vi "Doktorarbeit_Cornelius_1.8.vi"(0 "Heizer":refnum<visa-resource-name>="COM1", 1 "Setpoint\n START":bool, 2 "Write to File":bool, 3 "SP 1 shall be (°C)":dbl=20.0 min=0.0 max=999.0, 4 "Intervall (s)":u32=1 max=600, 5 "Write/\nRead":bool=TRUE, 6 "Delay (ms)":u32=500 min=100 max=600000, 7 "Auto Tune":bool, 9 "Standby":bool, 11 "Reset\nSTOPP":bool, 12 "ON":bool=TRUE caption="OFF", 13 "Get Values":bool, 15 "File Path":path) -> (8 "(°C)":dbl format="%#.3f", 14 "SP 1 is (°C)":dbl)   [LabVIEW 2010]
doc: "1. Verwendung\n\nDas Programm dient der Steuerung und Abfrage des Thermocontrollers I3252 und dem Auslesen von zwei VC 840 Messgeräten und einem Druckmessgerät Pfeiffer Single Gauge. \nDie Messgeräte werden Standardmäßig ausgelesen und erst nach Betätigung des Schalters \"Write to File\" in einer Textdatei abgespeichert. Das Eingabefeld \"Intervall\" legt den Abstand der Messpunkte fest.\nDer Setpoint für den Thermocontroller wird erst nach Betätigung des Tasters \"Setpoint START\" übernommen und angesteuert. Er wird ind den EEPROM des Gerätes geschrieben. Die Regelung kann mit Hilfe des Schalters \"Standby\" unterbrochen werden. Durch den Taster \"Reset STOPP\" kann der Setpoint aus dem EEPROM gelöscht werden.\nDie Eingabeflächen \"Constant\" und \"Thickness\" dienen der Berechnung des spezifischen Widerstands.\nDie Eingabeflächen \"User\" und \"Sample\" werden in den Header der Textdatei übernommen.\nDer Indikator \"File Path\" zeigt den aktuellen Speicherort der Textdatei an. Dieser wird nach ausschalten des Schalters \"Write to File\" gelöscht. Bei erneuten Schreiben muss ein neuer Speicherort gewählt werden. Bei Wahl desselben Speicherorts werden sämtliche bereits gespeicherte Daten gelöscht.\n\n\n2. Erläuterungen zum Blockdiagramm\n2.1 äußere Sequenz\nDie äußerte Sequenz besteht aus fünf Frames. Der erste dient der Initialisierung der Ports. Der zweite dient als Verzögerung um dem Programm genug Zeit zu geben die Ports zu öffnen. Jedoch senden die beiden VC 840 bereits Informationen an den Computer die in einem Puffer zwischengespeichert werden. Im dritten Frame wird dieser Puffer geleert. Somit kommt es zu keinem Framing Error. Desweiteren wird in diesem Frame die Startzeit der Messungen genommen. Im vierten Frame wird die eigentliche Messung und Verarbeitung der Daten durchgeführt. Die while-Schleife wird nur durch Auftreten eines Fehlers oder durch Betätigung des Stopbuttons auf dem Front Panel in der oberen linken Ecke unterbrochen. Im fünften und letzten Frame werden die Ports wieder geschlossen und beim Auftreten eines Fehlers wird das Programm automatisch gestoppt. Falls kein Fehler auftritt wird die Sequenz von vorne abgearbeitet.\n\n2.2 while-Schleife und innere Sequenz\n2.2.1 \"Event Structure\"\n2.2.1.1 Allgemein\nDer erste Frame beinhaltet ein \"Event Structure\". Dieser reagiert auf insgesamt elf verschiedene Ereignisse. Falls keines dieser Ereignisse auftreten sollte, warte die Struktur eine Millisekunde bevor die \"Event Structure\" verlassen wird. Die übrigen Ereignisse treten ein, wenn der entsprechende Kontroller eine Werteänderung erfährt.\n\n2.2.1.2 Event: Setpoint\nDieser Case besteht von außen nach innen aus einer Stacked Sequence, einer for-Loop und einer Flat Sequence die wiederum zwei \"Case Structures\" enthält. Als erstes wird bei dem Schalter \"Setpoint START\" der Blinkmodus aktiviert und bei dem Schalter \"Read Temperature\" deaktiviert. Danach folgt das eigentliche setzen des Temperatursollwerts. In der ersten Iteration wird dem Controller I3252 ein Schreibbefehl gesendet. Theoretisch kann der Setpoint in den RAM oder in den EEPROM geschrieben werden. Diese Auswahl erfolgt mit Hilfe des Schalters \"RAM\". Da das Schreiben in den RAM -Speicher aber aus diversen Gründen nicht erwünscht ist, wurde es nicht implementiert. Eine nachträgliche Implementierung ist aber leicht möglich, in dem die untere String-Konstante \"*P012\" durch \"*W012\" ersetzt wird. An diesem Befehl wird eine fünfstellige Hexadezimalzahl angehängt, die den Sollwert wiedergibt. Der Sollwert wird vorher mit zehn multipliziert, da das Komma standardmäßig nach der ersten Ziffer festgesetzt wurde (Bsp.: 800 wird gesendet um 80 einzustellen). Dieser Befehlsstrang wird an das Gerät mittels des SubVIs \"Comm_Interface\", auf welches später noch näher eingegangen wird, weitergegeben. Der durch das Gerät zurückgegebene String wird nicht verarbeitet.\nDie zweite Iteration dient dem Auslesen des eingestellten Sollwertes. Wahlweise kann der RAM- oder der EEPROM-Speicher ausgelesen werden. Die eigentliche Verarbeitung des Ausgabestrings erfolgt durch das SubVI \"Edit Setpoint\".\nDie Implementierung zur Einstellung des zweiten Setpoints erfolgt durch kopieren der ersten beiden Fälle und ersetzen der \"1\" im Befehf durch eine \"2\" (Bsp.: \"*P012\" zu \"*P022\"). Es darf aber nicht vergessen werden, dass dann ebenfalls die Anzahl der Iterationen angepasst werden muss.\nAls letztes wird der Blinkmodus des Schalters \"Setpoint START\" wieder deaktiviert.\n\n2.2.1.3 Event: Standby\nDieses Ereignis aktiviert bzw. deaktiviert als erstes den Blinckmodus des entsprechenden Schalters und sendet danach den Befehl zum aktivieren (\"*D03\") oder zum deaktivieren (\"*E03\") des Standbymodus an den Thermocontroller.\n\n2.2.1.4 Event: Set Command \nDer in das Feld \"Command shall be\" eingegebene Befehl wird an den Thermocontroller übermittlet. Die korrekte Form des Befehls ist im \"Communication Manuel\" nachzuschlagen. Das \"*\"-Zeichen wurde allerdings schon implementiert und muss somit nicht mit eingegeben werden.\n\n2.2.1.5 Event: Reset\nIn der ersten Iteration wird der Reset-Befehl an den Thermocontroller gesendet. In Folge wird der gesamte EEPROM-Speicher gelöscht. Deshalb wird in der zweiten Iteration der Setpoint aktualisiert. Dieser Befehl hat keinen Einfluss auf den RAM-Speicher. Die anschließende Wartezeit ist auf vier Sekunden festgesetzt und wurde empirisch ermittelt. Diese Zeit benötigt das Gerät um den Reset durchzuführen und für die Kommunikation wieder zur Verfügung zu stehen.\n\n2.2.1.6 Event: Auto Tune\nEs ist festgeschrieben, dass der Setpoint für die \"Auto Tune\"-Funktion wenigstens 20°C über der aktuellen Temperatur liegt. Deshalb wird zunächst der aktuelle Temperaturwert ausgelesen. Im zweiten Schritt werden zu diesem Wert zwanzig addiert und der Setpoint wird in den RAM-Speicher geschrieben. Das Schreiben in diesen Speicher ist nötig, da die \"Auto Tune\"-Funktion\" erst nach einem Reset startet. Im dritten Schritt wird der eigentliche Befehl für den \"Auto Tune\" gesendet (siehe dazu \"Communication Manuel\" S.27). Als vierte und letzte Iteration der for-Schleife folgt der bereits erwähnte Reset-Befehl. Der Temperatursollwert, der im RAM-Speicher eingetragen ist, muss zum Schluss wieder auf 0°C gesetzt werden. Die Zeit für die Ausführung des \"Auto Tune\"-Befehls wurde empirisch ermittelt und 45 s festgesetzt.\n\n2.2.1.7 Event: Write LOW/HI\nDieses Ereignis setzt die am Analogausgang anliegende Spannung fest. Normalerweise beträgt dieser Spannungswert 0-10 V. Das angeschlossene Netzteil verträgt aber maximal nur 2,3 V. Aus diesem Grund wird der \"%HIGH\" auf 23 gesetzt. Somit beträgt die maximal anliegende Spannung nur noch 23% von der maximal möglichen, d.h 2,3V. Ein niedrigerer Wert ist jederzeit möglich, genauso wie ein höherer für den Parameter \"%LOW\". Diese werden zunächst nacheinander in den RAM-Speicher geschrieben und anschließend wieder ausgelesen.\n\n2.2.1.8 Event: Set PID\nDie Werte für den PID-Regler können sowohl mit Hilfe der \"Auto Tune\"-Funktion, als auch manuell eingestellt werden. Es wird wiederum zwischen dem Schreiben in den RAM- und dem EEPROM-Speicher unterschieden. Zunächst werden die Werte für \"P\", \"I\" und \"D\", in dieser Reihenfolge, gesetzt und danach die aktuellen Werte ausgelesen.\n\n2.2.1.9 Event: Get Values\nDieses Ereignis hat zur Folge, dass die Werte für \"P\", \"I\", \"D\", \"%LOW\", \"%HIGH\" und des Setpoints wahlweise aus dem RAM- oder EEPROM-Speicher gelesen werden. Die aktuellen Werte werden nicht nur in die entsprechenden Anzeigefelder übernommen, sondern auch in die entsprechenden Eingabefelder, mit Ausnahme des Temperatursollwerts. \n\n2.2.1.10 Event: RAM\nPrinzipiell kann zwischen dem Schreiben in den RAM- oder EEPROM-Speicher des Thermocontrollers gewählt werden. Die entsprechende Schalterposition auf dem Frontpanel zeigt den aktuell verwendeten Speicher an. Die Anzeigewerte werden bei jedem Umschalten aktualisiert und sind im entsprechenden Speicher eingetragen. Die Implementierung ist identisch mit der des Ereignisses \"Get Values\". Es gilt zu beachten, dass die Werte für \"%LOW\" und \"%HIGH\" nur in den RAM-Speicher geschrieben werden können und somit auch nur aus diesem ausgelesen werden können.\n\n2.2.1.11 Event: Set Gauge to Zero\nMit Hilfe der SubVIs \"Get Pressure\" und \"Offset Display\" werden die Werte für den alten und den neuen Offset und der durch den zweiten Drucksensor ermittelt Druck ermittelt. \n\n2.2.1.12 Event: Write to File\nSollte der Schalter \"Write to File\" aktiviert werden, d.h. Schalterposition oben, so wird zunächst durch das SubVI \"Header\" ein Header für die unter \"File Path\" definierte Datei angelegt. Alle Werte, die bereits in der entsprechenden Datei stehen, werden dabei gelöscht.\n\n2.2.2 \"Timed Structures\"\nIm dritten Frame der inneren Sequenz werden die Werte für Zeitpunkt, Temperatur, Spannung, Strom und Druck ermittelt. Damit die Werte zum gleichen Zeitpunkt aufgenommen werden, werden \"Timed Sequences\" eingesetzt. Mit dem entsprechenden Schalter auf dem Front Panel unter dem Tab \"Settings\" kann gewählt werden, ob das entsprechende Gerät ausgelesen werden soll oder nicht. Die einzelnen Sequenzen werden parallel abgearbeitet, womit die Prozesszeit von diesem Frame durch der zeitintensivsten Sequenz abhängt. Dies ist in aller Regel das Auslesen der Temperatur, da ein \"Delay\" von 500 ms oder größer benötigt wird, um den Controller ordentlich ansprechen zu können.\nDie Systemzeit wird durch das SubVI \"System Time in Seconds\" in Sekunden umgerechnet und der in dem Parameter \"Starttime\" gespeicherte Wert wird abgezogen. Somit werden die Sekunden seit dem Start des Programms gezählt.\n\n2.2.3 restlichen Frames\nIm zweiten Frame wird das Intervall zwischen den einzelnen Messwerten festgelegt. Dabei wird der Wert des Parameters \"Delay\" abgezogen. Dieser Wert beträgt im Normalfall 500 ms und ist somit nicht vernachlääsigbar.\nDer Vierte Frame beinhaltet die Umrechnung des Temperatur-Strings in einen Temperaturwert durch das SubVI \"Edit Tmperature\", die Berechnung des spezifischen Widerstands durch das SubVI \"Resistivity Calculation\" und die Überprüfung des Druckwerts. Auch werden die neu gewonnen Werte in das entsprechende Shift-Register übernommen. Falls der Druckwert einen in dem Parameter \"Pressure Limit (mbar)\" festgelegten Grenzwert überschreiten sollte, wird der Thermocontroller automatisch in den Standby-Modus versetzt. Des Weiteren wird der Schalter \"Standby\" solange gesperrt, wie der Druck oberhalb des Grenzwertes liegt. Wenn der Druck wieder unter den Grenzwert gesunken ist, wird der Standby-Befehl nicht automatisch aufgehoben, sondern muss vom Benutzer durch Betätigung des entsprechenden Schalters gegeben werden.\nIm fünften Frame werden die Diagramme erstellt. Dabei wird jedes Mal von neuem das gesamte Shift-Register als Graph dargestellt. Weiterhin werden die Messwerte in ein 1D-Array geschrieben.\nDer sechste und letzte Frame beinhaltet den eigentlich Schreibvorgang der Messwerte in eine Textdatei und die Überprüfung ob ein Fehler vorliegt.\n\n2.3 SubVIs\n2.3.1 Allgemein\nDie SubVIs für die Messgeräte VC840 und das Druckmessgerät wurden aus anderen Quellen übernommen. \n\n2.3.2 \"Header\"\nIn den Header wird zunächst das aktuelle Datum und die aktuelle Zeit übernommen. Die ausgewählte Datei wird dabei überschrieben. Danach wird der Name des Benutzers und der Probe übernommen. Zum Schluss werden die Einheiten in einer Reihe, durch einen Tabulator getrennt, in den Header geschrieben.\n\n2.3.3 \"I3252 Comm Interface\"\nDieses VI stellt die Kommunikation mit dem Thermocontroller her und gibt den Ausgabe-String zurück.\n\n2.3.4 \"I3252 Edit Setpoint\"\nIm Ausgabe-String vom Thermocontroller ist an der vierten Stelle die Stelle des Dezimalpunktes verschlüsselt. Dieses Hexadezimalzahl wird herausgefiltert und an ein \"ENUM Controller\" übergeben. Dieser weist der Hexadezimalzahl eine Nummer zu, mit welcher ein Wert aus einem Array entnommen wird. Dieser Wert dient als Quotient. Der tatsächliche Wert kann somit errechnet werden.\n\n2.3.5 \"I3252 Edit Temperature\"\nDer Temperatur-String, der vom Thermocontroller zurückgegeben wird, wird in eine Dezimalzahl umgewandelt. Manchmal kommt es aus zu Dropouts, die durch dieses Programm herausgefiltert werden. Der letzte Wert wird dabei in einer \"Feedback Node\" gehalten unter der Annahme, dass sich der Temperaturwert nicht sprunghaft ändert.\n\n2.3.6 \"Resistivity Calculation\"\nDer spezifische Widerstand wird nach folgender Formel ausgerechnet. Dabei entspricht t der Dicke der Probe und C ist eine Konstante.\nrho=C*pi*t*U/(ln( 2)*I)\n\n2.3.7 \"System Time in Seconds\"\nZunächst wird die aktuelle Systemzeit ausgelesen. Danach wird diese in Stunden, Minuten und Sekunden aufgeteilt, alles in Sekunden umgerechnet und letztendlich addiert."
uses:
  <vilib>/Platform/TimedLoop/XDataNode/XDataNode.xnode
  <vilib>/Platform/TimedLoop/XDataNode/timing_clust.ctl
  <vilib>/Platform/TimedLoop/XDataNode/nitl_modes.ctl
  <vilib>/Platform/TimedLoop/XDataNode/wakeup.ctl
  <vilib>/Instr/_visa.llb/VISA Configure Serial Port (Instr).vi
  <vilib>/Platform/TimedLoop/scheduler/LVUserAPI/_suppVIs/Create_1kHz_TSource.vi
  <vilib>/Utility/file.llb/Write To Spreadsheet File (DBL).vi
  <vilib>/Platform/TimedLoop/XDataNode/XDNodeRunTimeDep.lvlib
  Labview 8 Tutorial/Dual Gauge/Dual Gauge.lvlib
panel:
  in  "Delay (ms) 2":u32=500 min=100 max=600000
  in  "Write/\nRead 2":bool=TRUE
  in  "Flow Control 2":u16(ring) items=["None"=0, "XON/XOFF"=1, "RTS/CTS"=2, "DTR/DSR"=4]
  in  "Stop Bits 2":u16(ring)=10 items=["1.0"=10, "1.5"=15, "2.0"=20]
  in  "Parity 2":u16(ring)=1 items=["None", "Odd", "Even", "Mark", "Space"]
  in  "Data Bits 2":u16=7 min=5 max=8 step=1
  in  "Baud Rate 2":u32=9600
  in  "Heizer 2":refnum<visa-resource-name>="COM1"
  out "appended array":dbl[](array[numeric])
  in  "Tab Control":T1(tab)
  out "Pirani (VVP1 Scroll)":cluster{dbl[], dbl[]}(graph)
  in  "Thickness (nm)":dbl min=0.0
  in  "Constant":dbl=4.532 min=0.0 max=5.0
  in  "Sample":string
  in  "User":string
  out "Thermocouple (Sample holder 1)":cluster{dbl[], dbl[]}(graph)
  out "current time (s)":dbl
  out "data logger intervall (s)":dbl
  out "loop time (s)":dbl
  in  "stop":bool
  out "CMR275 Baratron":cluster{dbl[], dbl[]}(graph)
  out "Pressure Baratron 2":dbl format="%#_4e"
  out "PKR251 FullRange":cluster{dbl[], dbl[]}(graph)
  out "Pressure FullRange 2":dbl format="%#_3e"
  out "Pressure Pirani 2":dbl format="%#_3e"
  out "Pressure OpenPort":cluster{dbl[], dbl[]}(graph)
  out "Pressure OpenPort2":dbl caption="current"
  out "status 2":bool caption="Status"
  out "code 2":i32 caption="Code"
  out "code":i32 caption="Code"
  out "status":bool caption="Status"
  in  "Set Gauge to Zero":bool
  out "Status Gauge 1#2":i32(ring) items=["data OK", "underrange", "overrange", "sensor error", "sensor off", "no sensor", "ID error"]
  out "Pressure Gauge 1#2":dbl format="%.3e"
  out "Pressure Gauge 1#1":dbl format="%.3e"
  out "Status Gauge 1#1":i32(ring) items=["data OK", "underrange", "overrange", "sensor error", "sensor off", "no sensor", "ID error"]
  in  "TPG 1 COM":refnum<visa-resource-name>="COM5"
  in  "Pressure Limit (mbar)":dbl=1.0 min=0.0 max=1100.0
  out "Current Offset (mbar)":dbl
  in  "ON (TPG 2)":bool=TRUE caption="OFF"
  in  "ON (TPG 1)":bool=TRUE caption="OFF"
  in  "ON":bool caption="OFF"
  in  "VC 840 2":refnum<visa-resource-name>="COM7"
  out "Reading 2":dbl format="%_4f"
  out "Mode 2":enum16{"?", "Diode", "Beep", "DC", "AC"}(ring)
  out "Unit 2":string
  in  "VC 840 1":refnum<visa-resource-name>="COM7"
  out "Reading 1":dbl format="%_4f"
  out "Mode 1":enum16{"?", "Diode", "Beep", "DC", "AC"}(ring)
  out "Unit 1":string
  out "Status 1":T2
  out "Status 2":T2
  in  "ON":bool caption="OFF"
  out "% HIGH Istwert":u32
  out "% LOW Istwert":u32
  in  "% High Sollwert":u32=23 max=24
  in  "% LOW Sollwert":u32 max=25
  in  "RAM":bool=TRUE caption="EEPROM"
  out "D (Rate) IstWert":u32
  out "I ( Reset1) Istwert":u32
  out "P (PB1) Istwert":u32 caption="actual value"
  in  "D (Rate) Sollwert":u32 max=3999
  in  "I ( Reset1) Sollwert":u32 max=3999
  in  "P (PB1) Sollwert":u32 caption="set value" max=9999
  in  "Set Command":bool
  in  "Set PID":bool
  in  "Write LOW/HI":bool
  in  "Flow Control":u16(ring) items=["None"=0, "XON/XOFF"=1, "RTS/CTS"=2, "DTR/DSR"=4]
  in  "Stop Bits":u16(ring)=10 items=["1.0"=10, "1.5"=15, "2.0"=20]
  in  "Parity":u16(ring)=1 items=["None", "Odd", "Even", "Mark", "Space"]
  in  "Data Bits":u16=7 min=5 max=8 step=1
  in  "Baud Rate":u32=9600
  out "Command output":string
  in  "Command input":string
  in  "TPG 2 COM":refnum<visa-resource-name>="COM6"
  out "Pressure Gauge 2#2":dbl format="%.3e"
  out "Pressure Gauge 2#1":dbl format="%.3e"
  out "Status Gauge 2#2":i32(ring) items=["data OK", "underrange", "overrange", "sensor error", "sensor off", "no sensor", "ID error"]
  out "Status Gauge 2#1":i32(ring) items=["data OK", "underrange", "overrange", "sensor error", "sensor off", "no sensor", "ID error"]
  out "Current":cluster{dbl[], dbl[]}(graph)
  out "Voltage":cluster{dbl[], dbl[]}(graph)
  out "Voltage (V)":dbl format="%.4e"
  out "Current (A)":dbl format="%.4e"
  out "Resistivity":cluster{dbl[], dbl[]}(graph)
  out "Resistivity (Ohm*cm)":dbl format="%.3e"
  # "mbar"
  # "mbar"
  # "mbar"
  # "mbar"
  # "Pressure Measurement \n(Pfeiffer TPG261)"
  # "PID Controller (Omega Newport i3252)"
  # "PID Controller (Omega Newport i3252)"
  # "limit (mbar)"
  # "Multimeter\n#1 (VC 840)"
  # "Multimeter\n#2 (VC 840)"
  # "P"
  # "I"
  # "D"
  # "% Low"
  # "% High"
  # "Authors:  Daniel Schuster (sir-dan@web.de)\n                 Steffen Cornelius (s.cornelius@hzdr.de)\n                 Nico Spahn (x)\n\n                 premade SubVIs for readout of Pfeiffer gauge and VC840 Multimeters were used\n                 SubVI \"I3252_Comm_Interface\" is based on a modified Labview example\n\nRelease:  v1.0    \n\nVersion History:\n\nv1.1  -    28.06.2011\n             - Format des Files geändert von %.3f auf %g\n             - maximale Eingabewerte für PID begrenzt\nv1.2  -    12.07.2011\n             - Anzeige p,rho, U, V auf Scientific geändert\n             - y-Achse p,rho auf Log geändert\n             - numerische Zeitanzeige hinzugefügt\n             - 4PP Constant: pi/ln(2)=4,532 set as the default value\nv1.3  -    25.07.2011\n             - Zeitvariable auf EXT geändert, um Sprünge in Diagrammen loszuwerden\nv1.4  -   27.07.2011\n             - ALLE Variablen auf DBL zurückgesetzt wegen Formatierungsproblem im File\n             - Zeitberechnung neu gemacht (Tick count differenzen) -> Zeitsprünge korrigiert ?\n             - Delay/Intervall überarbeitet\nv1.5  -   05.12.2012\n                - Austausch der alten Pfeifer SubvIs durch neue -> nun alle 4 Kanäle des DualGauge\n                                                                                                         Controllers gleichzeitig auslesbar\n                - neue Pfeiffer SubVIs verwendet in Druckwertauslesung und Offset Berechnung des Baratron\n                  Druckes (COM5 Sensor1)\n                - Neuarragement des GUI -> FullRange und Baratron neben Temperatur auf Haupseite zu sehen\n                                                                   Pirani und OpenPort auf Meas.2 zu sehen\n                                                                   Diagnose Seite umfasst nun auch Widerstandsdiagramm\n                - Änderungen der Settingseite -> nun alle 4 Drucksensoren mit aktuellem Messwert und Gerätestatus\n                                                                           zu sehen\n                - The readout of the PID-Temperature Controller and the VC840 Multimeters was not modified\nv1.73  -  18.10.2013\n                - Layout Änderungen\nv.1.8   -  19.01.2014\n                - Änderung Layout Settings Tab\n                - Trennung der beiden TPG Dual Gauge Controls\n                -"
  # "Version 1.73    - last change 18.10.2013"
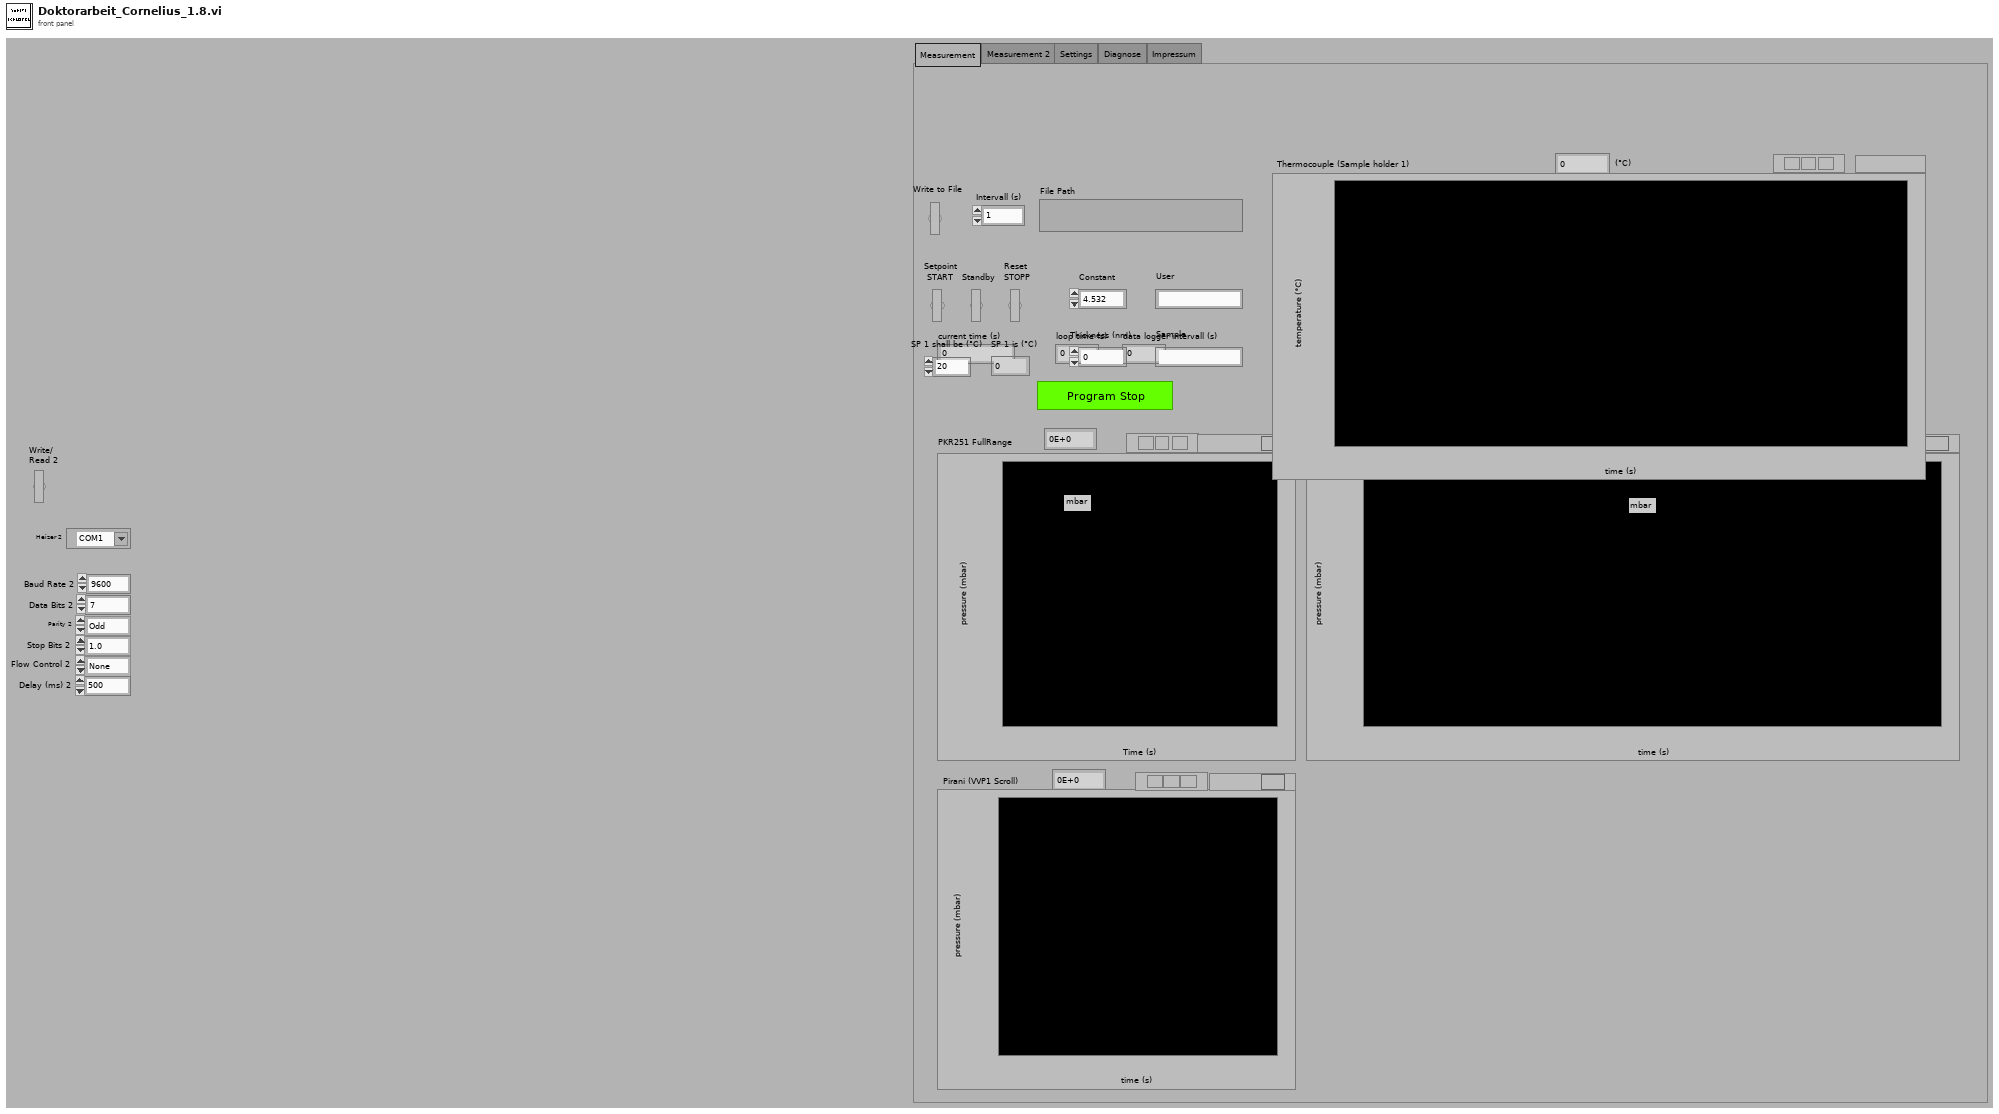
[diagram p1: front panel]
types:
  T1 = enum32{"Measurement", "Measurement 2", "Settings", "Diagnose", "Impressum"}
  T2 = cluster{"Low Bat":bool, "Auto":bool, "Delta":bool, "Hold":bool, "RS232":bool}
  T3 = typedef "XDNodeRunTimeDep.lvlib/timing_clust.ctl" = cluster{"Expected End [f-1]":u64, "Actual End [f-1]":u64, "Finished Late? [f-1]":bool, "Expected End [i-1]":u64, "Actual End [i-1]":u64, "Finished Late? [i-1]":bool, "Expected Start [i]":u64, "Actual Start [i]":u64, "Expected Start [f]":u64, "Actual Start [f]":u64, "Source Name":string, "Structure Name":string, "Period":i64, "Deadline":i64, "Offset":i64, "Start":i64, "Priority":i32, "Timeout":i32, "Mode":T4, "Wakeup Reason":T5, "Error":errorcluster, "Source Type":string, "Secondary Source Type":string, "Global End Time":u64, "Global Start Time":u64, "Frame Duration":u64, "Iteration Duration":u64, "Assigned CPU":i32, "I/O Scan Engine Mode":u32}
  T4 = typedef "XDNodeRunTimeDep.lvlib/nitl_modes.ctl" = enum32{"No Change", "Process missed periods, maintain original phase", "Discard missed periods, maintain original phase", "Process missed periods, ignore original phase", "Discard missed periods, ignore original phase"}
  T5 = typedef "XDNodeRunTimeDep.lvlib/wakeup.ctl" = enum32{"Normal", "Aborted", "Asynchronous wakeup", "Timing source error", "Timed loop error", "Timeout"}
  T6 = enum8{"Enabled", "Disabled", "Disabled and Grayed Out"}
  T7 = cluster{"VISA resource name out":refnum<visa-resource-name>, "error out":errorcluster, "Delay (ms)":u32, "Write/\nRead":bool}
  T8 = cluster{"TPG 2 COM":refnum<visa-resource-name>, "error out":errorcluster}
  T9 = cluster{"COM out":refnum<visa-resource-name>, "Cluster (Ausgang)":errorcluster}
  T10 = cluster{"Pressure Gauge#1":dbl, "Pressure Gauge#2":dbl}
  T11 = cluster{"TPG 1 COM":refnum<visa-resource-name>, "error out":errorcluster}
  T12 = cluster{"COM out":refnum<visa-resource-name>, "error out":errorcluster, "COM out":refnum<visa-resource-name>, "error out":errorcluster}
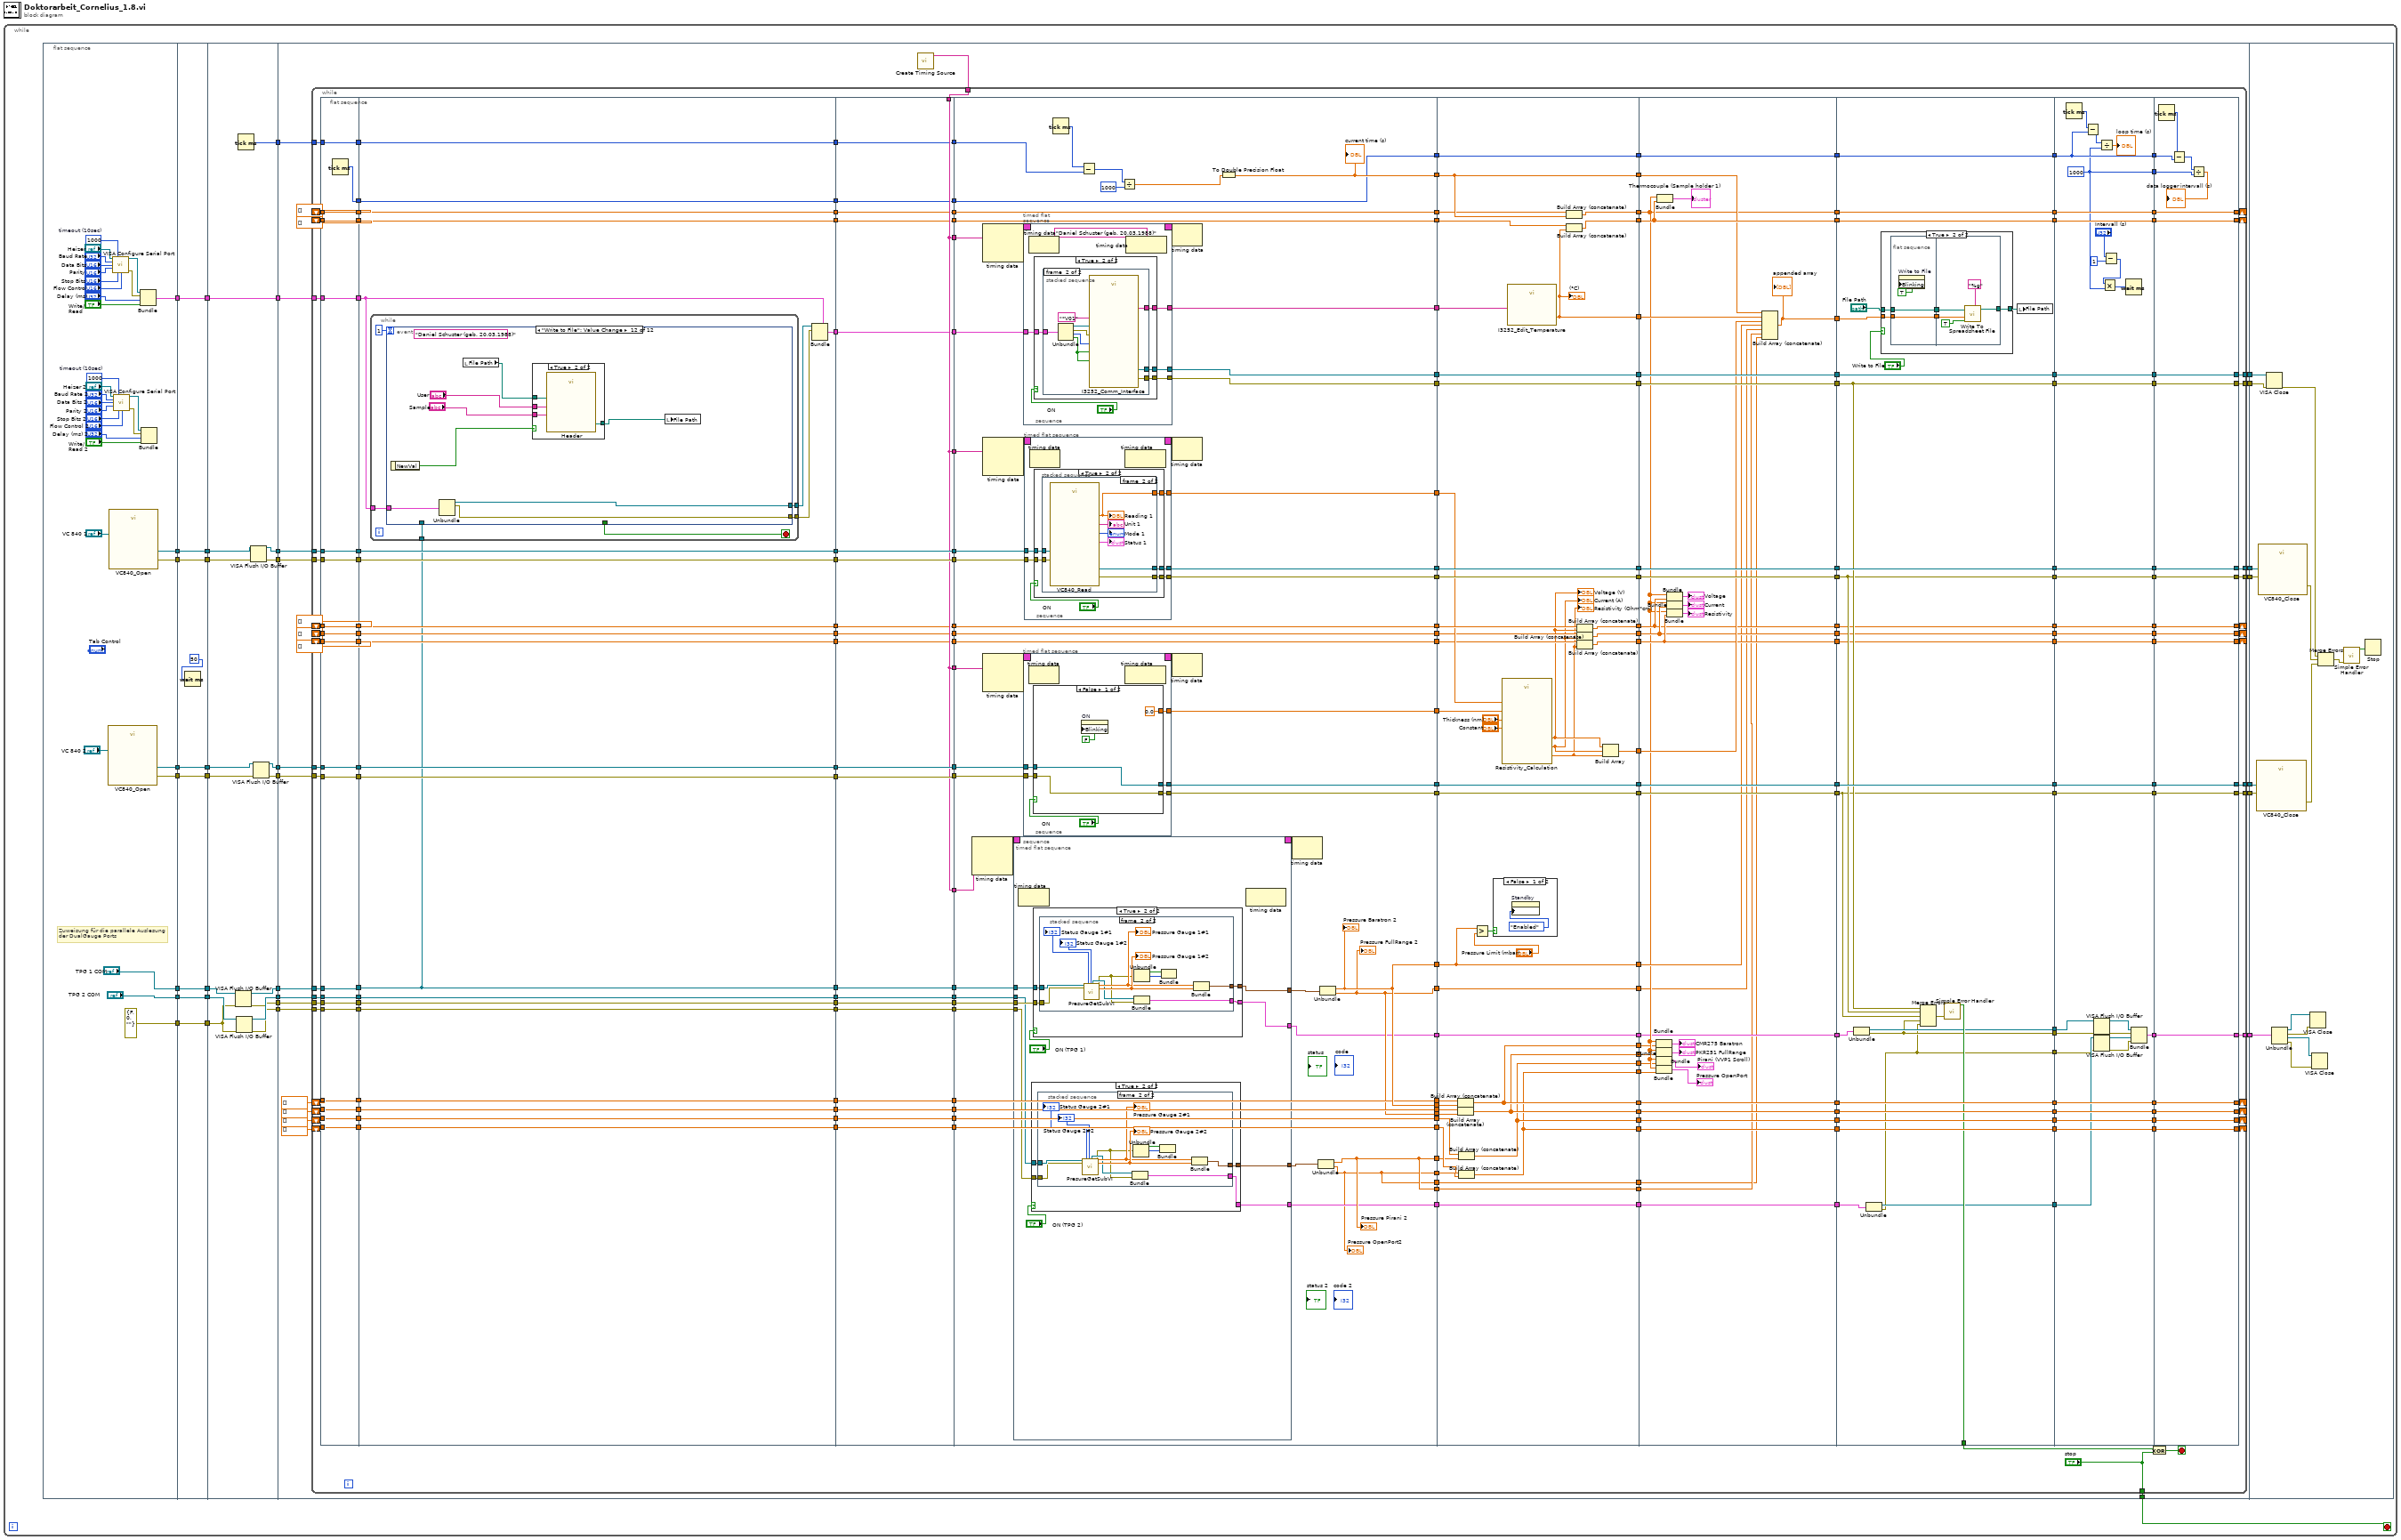
[diagram p0: block diagram]
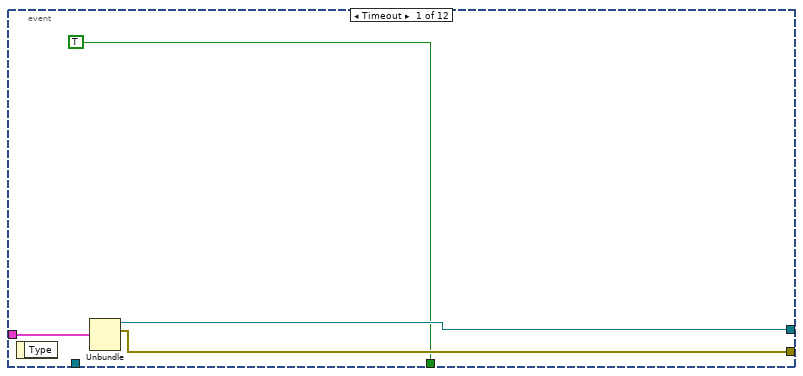
[diagram p2: hidden frame]
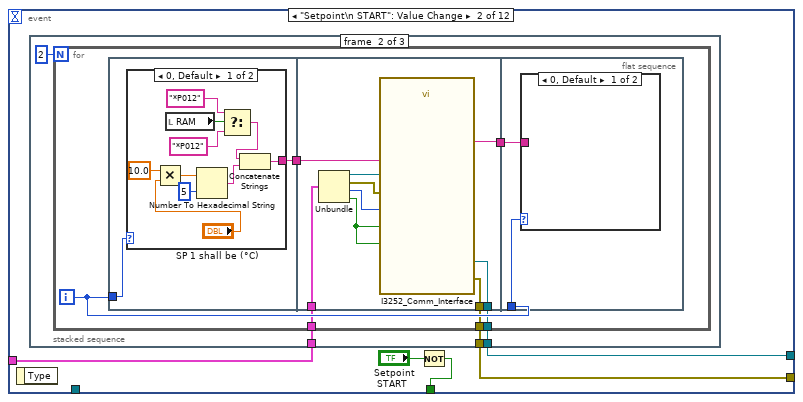
[diagram p3: hidden frame]
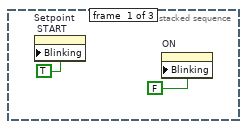
[diagram p4: hidden frame]
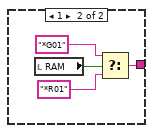
[diagram p5: hidden frame]
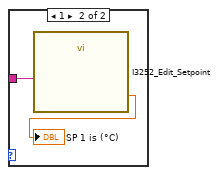
[diagram p6: hidden frame]
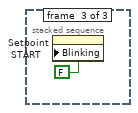
[diagram p7: hidden frame]
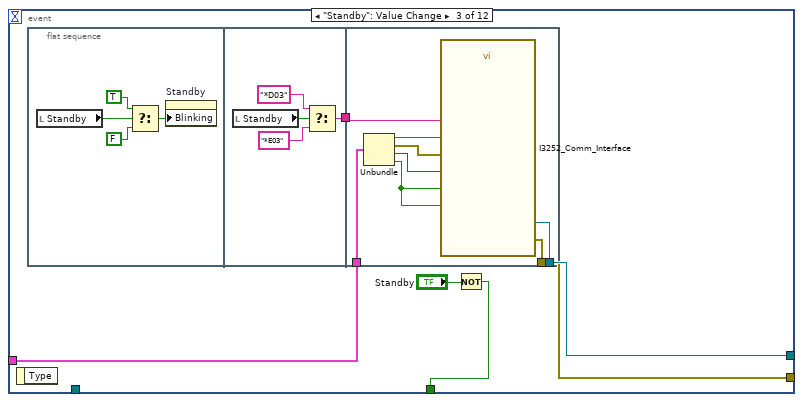
[diagram p8: hidden frame]
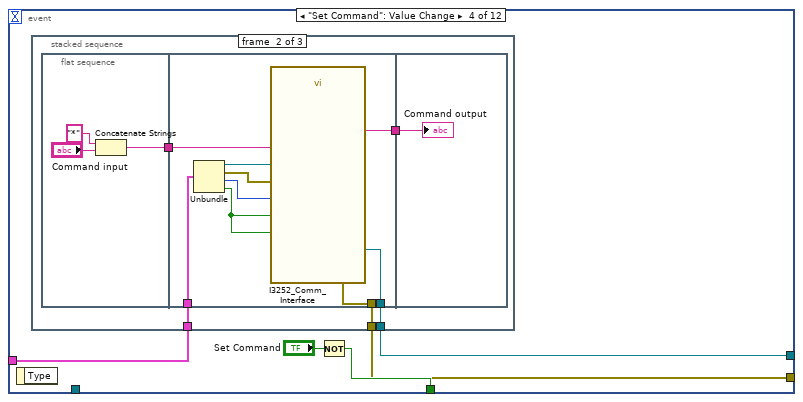
[diagram p9: hidden frame]
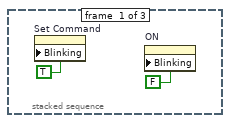
[diagram p10: hidden frame]
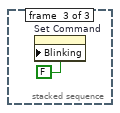
[diagram p11: hidden frame]
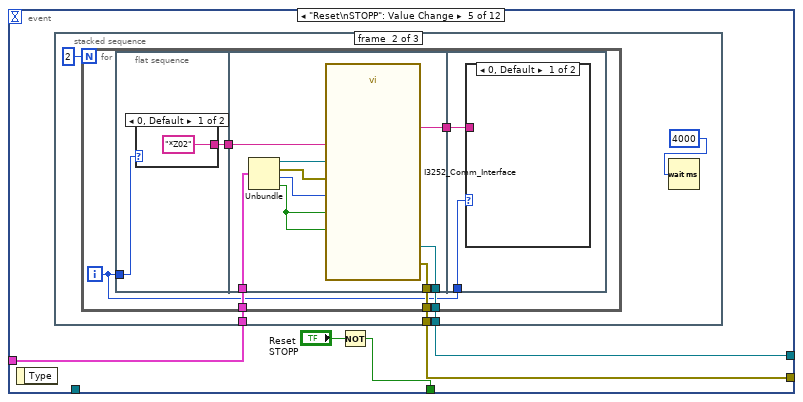
[diagram p12: hidden frame]
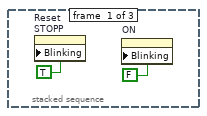
[diagram p13: hidden frame]
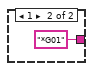
[diagram p14: hidden frame]
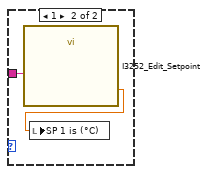
[diagram p15: hidden frame]
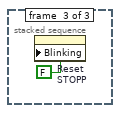
[diagram p16: hidden frame]
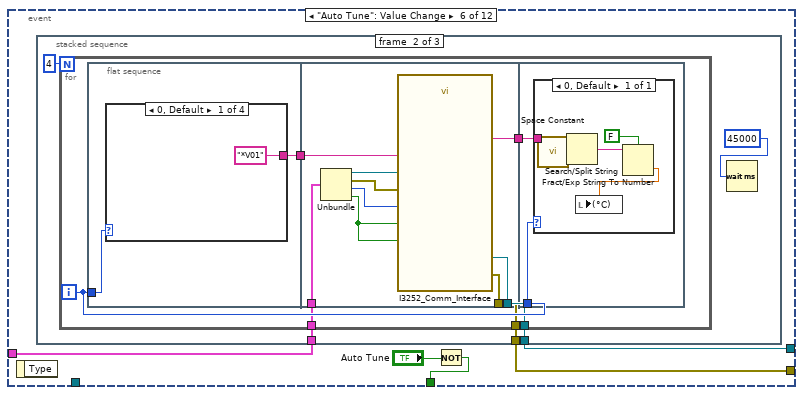
[diagram p17: hidden frame]
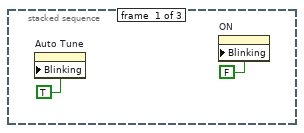
[diagram p18: hidden frame]
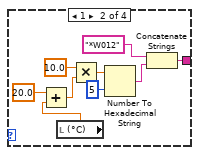
[diagram p19: hidden frame]
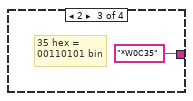
[diagram p20: hidden frame]
diagram:
  n1 = while {
    stop <- w6 stop-if-true
    n2 = flat-sequence {
      tunnel: [w65] -> w34
      tunnel: [w66] -> w33
      tunnel: [w51] -> w32
      tunnel: [w64] -> w31
      tunnel: [w63] -> w30
      tunnel: ["TPG 1 COM"] -> w29
      tunnel: ["TPG 2 COM"] -> w28
      tunnel: [errorcluster {"status"=FALSE, "code"=0, "source"=""} ("Fehler (Eingang)")] -> w3
      tunnel: w34 -> [w75]
      tunnel: [w75] -> w27
      tunnel: w33 -> [w74]
      tunnel: [w74] -> w26
      tunnel: w32 -> [w73]
      tunnel: [w73] -> w25
      tunnel: w31 -> [w72]
      tunnel: [w72] -> w24
      tunnel: w30 -> [w71]
      tunnel: [w71] -> w23
      tunnel: [w69] -> w22
      tunnel: w29 -> [w69]
      tunnel: [w68] -> w21
      tunnel: w28 -> [w68]
      tunnel: [w67] -> w4
      tunnel: w3 -> [w67]
      tunnel: w27 -> [w86]
      tunnel: [w85] -> w20
      tunnel: w26 -> [w87]
      tunnel: [w84] -> w19
      tunnel: w25 -> [w92]
      tunnel: [w92] -> w18
      tunnel: w24 -> [w89]
      tunnel: [w90] -> w17
      tunnel: w23 -> [w88]
      tunnel: [w91] -> w16
      tunnel: [w83] -> w15
      tunnel: [w81] -> w14
      tunnel: w22 -> [w82]
      tunnel: [w80] -> w13
      tunnel: w21 -> [w79]
      tunnel: w4 -> [w78]
      tunnel: [w77] -> w2
      tunnel: [w76] -> w1
      tunnel: w20 -> [w120]
      tunnel: w19 -> [w119]
      tunnel: w18 -> [w118]
      tunnel: w17 -> [w116]
      tunnel: w16 -> [w115]
      tunnel: [w114] -> w12
      tunnel: [w113] -> w11
      tunnel: [w112] -> w10
      tunnel: [w111] -> w9
      tunnel: [w110] -> w8
      tunnel: [w109] -> w7
      tunnel: w15 -> [w103]
      tunnel: w14 -> [w102]
      tunnel: w13 -> [w101]
      tunnel: [w96] -> w6
      tunnel: [w95] -> w5
      tunnel: w2 -> [w94]
      tunnel: w1 -> [w93]
      tunnel: w12 -> [w1327]
      tunnel: w11 -> [w1326]
      tunnel: w10 -> [w1329]
      tunnel: w9 -> [w1328]
      tunnel: w8 -> [w1331]
      tunnel: w7 -> [w1330]
      tunnel: w5 -> [w1324]
      frame #0 {
        w35 = u32 1000  # timeout (10sec)
        w52 = u32 1000  # timeout (10sec)
        # "Zuweisung für die parallele Auslesung\nder DualGauge Ports"
        n3 = call "VC840_Open.vi"("VISA resource name"="VC 840 2") -> ("error out"=w63:errorcluster, "VISA resource name out"=w64:refnum<visa-resource-name>)  [unwired: 1 in, 8 out]
        n4 = call "VC840_Open.vi"("VISA resource name"="VC 840 1") -> ("error out"=w66:errorcluster, "VISA resource name out"=w65:refnum<visa-resource-name>)  [unwired: 1 in, 8 out]
        n5 = call-poly "VISA Configure Serial Port"("VISA resource name"="Heizer", "timeout (10sec)"=w52, "baud rate (9600)"="Baud Rate", "data bits (8)"="Data Bits", "parity (0:none)"="Parity", "stop bits (10: 1 bit)"="Stop Bits", "flow control (0:none)"="Flow Control") -> ("VISA resource name out"=w61:refnum<visa-resource-name>, "error out"=w62:errorcluster)  [unwired: 2 in, 5 out]
        n6 = call-poly "VISA Configure Serial Port"("VISA resource name"="Heizer 2", "timeout (10sec)"=w35, "baud rate (9600)"="Baud Rate 2", "data bits (8)"="Data Bits 2", "parity (0:none)"="Parity 2", "stop bits (10: 1 bit)"="Stop Bits 2", "flow control (0:none)"="Flow Control 2") -> ("VISA resource name out"=w44:refnum<visa-resource-name>, "error out"=w45:errorcluster)  [unwired: 2 in, 5 out]
        n7 = Bundle("VISA resource name out"=w61, "error out"=w62, "Delay (ms)"="Delay (ms)", "Write/\nRead"="Write/\nRead") -> (w51:T7)  [unwired: 1 in]
        n8 = Bundle("VISA resource name out"=w44, "error out"=w45, "Delay (ms) 2"="Delay (ms) 2", "Write/\nRead 2"="Write/\nRead 2") -> ()  [unwired: 1 in, 1 out]
      }
      frame #1 {
        n9 = Wait (ms)(milliseconds to wait=u32 50) -> ()  [unwired: 1 out]
      }
      frame #2 {
        n10 = VISA Flush I/O Buffer(VISA resource name=w82, error in (no error)=w78) -> (VISA resource name out=w81:refnum<visa-resource-name>, error out=w77:errorcluster)  [unwired: 1 in]
        n11 = VISA Flush I/O Buffer(VISA resource name=w79, error in (no error)=w78) -> (VISA resource name out=w80:refnum<visa-resource-name>, error out=w76:errorcluster)  [unwired: 1 in]
        n12 = Tick Count (ms)() -> (millisecond timer value=w83:u32)
        n13 = VISA Flush I/O Buffer(VISA resource name=w86, error in (no error)=w87) -> (VISA resource name out=w85:refnum<visa-resource-name>, error out=w84:errorcluster)  [unwired: 1 in]
        n14 = VISA Flush I/O Buffer(VISA resource name=w89, error in (no error)=w88) -> (VISA resource name out=w90:refnum<visa-resource-name>, error out=w91:errorcluster)  [unwired: 1 in]
      }
      frame #3 {
        n15 = call-poly <vilib>:"Create Timing Source.vi"() -> ("name (out)"=w117:string)  [unwired: 10 in, 1 out]
        n16 = while {
          tunnel: w120 -> [w339]
          tunnel: w119 -> [w338]
          tunnel: w118 -> [w337]
          tunnel: w117 -> [w330]
          tunnel: w116 -> [w323]
          tunnel: w115 -> [w322]
          tunnel: [w318] -> w114
          tunnel: [w317] -> w113
          tunnel: [w315] -> w112
          tunnel: [w313] -> w111
          tunnel: [w311] -> w110
          tunnel: [w309] -> w109
          shift-right: [w282] -> _
          shift-left: dbl[] [] -> [w287]
          shift-right: [w260] -> _
          shift-left: dbl[] [] -> [w295]
          shift-right: [w284] -> _
          shift-left: dbl[] [] -> [w291]
          shift-right: [w257] -> _
          shift-left: dbl[] [] -> [w294]
          shift-right: [w254] -> _
          shift-left: dbl[] [] -> [w293]
          tunnel: w103 -> [w248]
          tunnel: w102 -> [w204]
          tunnel: w101 -> [w200]
          shift-right: [w158] -> _
          shift-left: dbl[] [] -> [w188]
          shift-right: [w156] -> _
          shift-left: dbl[] [] -> [w186]
          shift-right: [w154] -> _
          shift-left: dbl[] [] -> [w184]
          shift-right: [w152] -> _
          shift-left: dbl[] [] -> [w182]
          tunnel: ["stop"] -> w96
          tunnel: [w146] -> w95
          tunnel: w94 -> [w141]
          tunnel: w93 -> [w139]
          stop <- w145 stop-if-true
          n17 = flat-sequence {
            tunnel: w248 -> [w349]
            tunnel: w287 -> [w350]
            tunnel: w291 -> [w351]
            tunnel: w293 -> [w352]
            tunnel: w294 -> [w353]
            tunnel: w295 -> [w354]
            tunnel: w322 -> [w355]
            tunnel: w323 -> [w356]
            tunnel: w337 -> [w357]
            tunnel: w338 -> [w358]
            tunnel: w339 -> [w359]
            tunnel: [w359] -> w247
            tunnel: [w358] -> w246
            tunnel: [w357] -> w245
            tunnel: [w356] -> w244
            tunnel: [w355] -> w243
            tunnel: [w354] -> w242
            tunnel: [w353] -> w241
            tunnel: [w352] -> w240
            tunnel: [w351] -> w239
            tunnel: [w350] -> w238
            tunnel: [w349] -> w237
            tunnel: [w348] -> w219
            tunnel: [w347] -> w205
            tunnel: w204 -> [w347]
            tunnel: [w346] -> w201
            tunnel: w200 -> [w346]
            tunnel: [w345] -> w189
            tunnel: w188 -> [w345]
            tunnel: [w344] -> w187
            tunnel: w186 -> [w344]
            tunnel: [w343] -> w185
            tunnel: w184 -> [w343]
            tunnel: [w342] -> w183
            tunnel: w182 -> [w342]
            tunnel: [w341] -> w142
            tunnel: w141 -> [w341]
            tunnel: [w340] -> w140
            tunnel: w139 -> [w340]
            tunnel: [w382] -> w336
            tunnel: [w381] -> w334
            tunnel: [w377] -> w332
            tunnel: [w376] -> w327
            tunnel: [w375] -> w325
            tunnel: [w374] -> w292
            tunnel: [w373] -> w288
            tunnel: [w372] -> w268
            tunnel: [w371] -> w265
            tunnel: [w370] -> w263
            tunnel: [w369] -> w249
            tunnel: w247 -> [w382]
            tunnel: w246 -> [w381]
            tunnel: w245 -> [w380]
            tunnel: w244 -> [w376]
            tunnel: w243 -> [w375]
            tunnel: w242 -> [w372]
            tunnel: w241 -> [w371]
            tunnel: w240 -> [w370]
            tunnel: w239 -> [w374]
            tunnel: w238 -> [w373]
            tunnel: w237 -> [w369]
            tunnel: [w368] -> w220
            tunnel: w219 -> [w368]
            tunnel: w205 -> [w366]
            tunnel: [w366] -> w202
            tunnel: w201 -> [w367]
            tunnel: [w367] -> w198
            tunnel: w189 -> [w365]
            tunnel: w187 -> [w364]
            tunnel: w185 -> [w363]
            tunnel: w183 -> [w362]
            tunnel: [w365] -> w181
            tunnel: [w364] -> w177
            tunnel: [w363] -> w174
            tunnel: [w362] -> w173
            tunnel: w142 -> [w361]
            tunnel: w140 -> [w360]
            tunnel: [w361] -> w137
            tunnel: [w360] -> w135
            tunnel: w336 -> [w907]
            tunnel: [w907] -> w335
            tunnel: w334 -> [w906]
            tunnel: [w906] -> w333
            tunnel: w332 -> [w902]
            tunnel: [w902] -> w331
            tunnel: w330 -> [w903]
            tunnel: [w903] -> w329
            tunnel: [w903] -> w328
            tunnel: w327 -> [w905]
            tunnel: [w905] -> w326
            tunnel: w325 -> [w904]
            tunnel: [w904] -> w324
            tunnel: [w903] -> w321
            tunnel: [w903] -> w307
            tunnel: w292 -> [w901]
            tunnel: [w901] -> w290
            tunnel: w288 -> [w900]
            tunnel: [w900] -> w285
            tunnel: [w899] -> w269
            tunnel: w268 -> [w899]
            tunnel: [w898] -> w266
            tunnel: w265 -> [w898]
            tunnel: [w897] -> w264
            tunnel: w263 -> [w897]
            tunnel: [w896] -> w250
            tunnel: w249 -> [w896]
            tunnel: [w895] -> w221
            tunnel: w220 -> [w895]
            tunnel: [w894] -> w203
            tunnel: w202 -> [w894]
            tunnel: [w893] -> w199
            tunnel: w198 -> [w893]
            tunnel: w181 -> [w892]
            tunnel: [w892] -> w180
            tunnel: [w891] -> w178
            tunnel: w177 -> [w891]
            tunnel: [w890] -> w176
            tunnel: w174 -> [w890]
            tunnel: w173 -> [w889]
            tunnel: [w889] -> w172
            tunnel: [w888] -> w138
            tunnel: w137 -> [w888]
            tunnel: [w887] -> w136
            tunnel: w135 -> [w887]
            tunnel: [w930] -> w306
            tunnel: w335 -> [w959]
            tunnel: w333 -> [w958]
            tunnel: w331 -> [w955]
            tunnel: w329 -> [w954]
            tunnel: w328 -> [w953]
            tunnel: w326 -> [w943]
            tunnel: w324 -> [w942]
            tunnel: w321 -> [w944]
            tunnel: [w940] -> w305
            tunnel: [w941] -> w304
            tunnel: [w952] -> w303
            tunnel: [w951] -> w302
            tunnel: [w950] -> w301
            tunnel: [w949] -> w300
            tunnel: w307 -> [w939]
            tunnel: [w938] -> w299
            tunnel: [w937] -> w298
            tunnel: [w921] -> w297
            tunnel: [w936] -> w296
            tunnel: w290 -> [w935]
            tunnel: [w935] -> w289
            tunnel: [w934] -> w286
            tunnel: w285 -> [w934]
            tunnel: w269 -> [w933]
            tunnel: [w933] -> w267
            tunnel: w266 -> [w932]
            tunnel: w264 -> [w931]
            tunnel: [w932] -> w262
            tunnel: [w931] -> w261
            tunnel: w250 -> [w929]
            tunnel: [w925] -> w222
            tunnel: w221 -> [w925]
            tunnel: w203 -> [w923]
            tunnel: w199 -> [w922]
            tunnel: [w916] -> w197
            tunnel: [w921] -> w196
            tunnel: [w919] -> w195
            tunnel: [w917] -> w194
            tunnel: w180 -> [w920]
            tunnel: [w920] -> w179
            tunnel: w178 -> [w919]
            tunnel: w176 -> [w918]
            tunnel: [w918] -> w175
            tunnel: w172 -> [w917]
            tunnel: [w916] -> w150
            tunnel: [w915] -> w147
            tunnel: w138 -> [w914]
            tunnel: w136 -> [w913]
            tunnel: [w910] -> w131
            tunnel: [w908] -> w130
            tunnel: [w910] -> w129
            tunnel: [w909] -> w125
            tunnel: [w908] -> w122
            tunnel: w306 -> [w1169]
            tunnel: [w1166] -> w280
            tunnel: w305 -> [w1182]
            tunnel: [w1182] -> w279
            tunnel: w304 -> [w1181]
            tunnel: [w1181] -> w278
            tunnel: w303 -> [w1180]
            tunnel: [w1180] -> w277
            tunnel: w302 -> [w1179]
            tunnel: [w1179] -> w276
            tunnel: w301 -> [w1178]
            tunnel: [w1178] -> w275
            tunnel: w300 -> [w1177]
            tunnel: [w1177] -> w274
            tunnel: [w1170] -> w273
            tunnel: w299 -> [w1163]
            tunnel: w298 -> [w1171]
            tunnel: w297 -> [w1170]
            tunnel: w296 -> [w1172]
            tunnel: [w1169] -> w272
            tunnel: w289 -> [w1168]
            tunnel: w286 -> [w1167]
            tunnel: [w1165] -> w271
            tunnel: [w1153] -> w270
            tunnel: w267 -> [w1164]
            tunnel: w262 -> [w1161]
            tunnel: w261 -> [w1160]
            tunnel: [w1162] -> w258
            tunnel: [w1159] -> w255
            tunnel: [w1158] -> w252
            tunnel: [w1154] -> w251
            tunnel: [w1152] -> w223
            tunnel: w222 -> [w1152]
            tunnel: w197 -> [w1151]
            tunnel: w196 -> [w1150]
            tunnel: w195 -> [w1149]
            tunnel: w194 -> [w1147]
            tunnel: [w1145] -> w193
            tunnel: [w1144] -> w192
            tunnel: [w1143] -> w191
            tunnel: [w1142] -> w190
            tunnel: w179 -> [w1146]
            tunnel: w175 -> [w1148]
            tunnel: [w1145] -> w171
            tunnel: [w1144] -> w170
            tunnel: [w1143] -> w169
            tunnel: [w1142] -> w168
            tunnel: [w1141] -> w151
            tunnel: w150 -> [w1141]
            tunnel: [w1140] -> w148
            tunnel: w147 -> [w1140]
            tunnel: w131 -> [w1139]
            tunnel: w130 -> [w1138]
            tunnel: w129 -> [w1137]
            tunnel: [w1137] -> w128
            tunnel: [w1136] -> w126
            tunnel: w125 -> [w1136]
            tunnel: w122 -> [w1135]
            tunnel: [w1135] -> w121
            tunnel: w280 -> [w1216]
            tunnel: [w1223] -> w320
            tunnel: [w1222] -> w319
            tunnel: w279 -> [w1222]
            tunnel: [w1217] -> w316
            tunnel: w278 -> [w1217]
            tunnel: [w1221] -> w314
            tunnel: w277 -> [w1221]
            tunnel: [w1220] -> w312
            tunnel: w276 -> [w1220]
            tunnel: [w1219] -> w310
            tunnel: w275 -> [w1219]
            tunnel: [w1218] -> w308
            tunnel: w274 -> [w1218]
            tunnel: w273 -> [w1205]
            tunnel: w272 -> [w1206]
            tunnel: w271 -> [w1201]
            tunnel: [w1201] -> w283
            tunnel: w270 -> [w1207]
            tunnel: [w1207] -> w281
            tunnel: [w1209] -> w259
            tunnel: w258 -> [w1209]
            tunnel: [w1210] -> w256
            tunnel: w255 -> [w1210]
            tunnel: [w1211] -> w253
            tunnel: w252 -> [w1211]
            tunnel: w251 -> [w1215]
            tunnel: [w1204] -> w224
            tunnel: w223 -> [w1204]
            tunnel: w193 -> [w1200]
            tunnel: w192 -> [w1199]
            tunnel: w191 -> [w1198]
            tunnel: w190 -> [w1197]
            tunnel: w171 -> [w1196]
            tunnel: w170 -> [w1195]
            tunnel: w169 -> [w1194]
            tunnel: w168 -> [w1193]
            tunnel: [w1196] -> w166
            tunnel: [w1195] -> w164
            tunnel: [w1194] -> w162
            tunnel: [w1193] -> w160
            tunnel: w151 -> [w1192]
            tunnel: [w1191] -> w149
            tunnel: w148 -> [w1191]
            tunnel: w128 -> [w1188]
            tunnel: [w1187] -> w127
            tunnel: w126 -> [w1187]
            tunnel: w121 -> [w1186]
            tunnel: w320 -> [w1236]
            tunnel: w319 -> [w1251]
            tunnel: w316 -> [w1245]
            tunnel: w314 -> [w1250]
            tunnel: w312 -> [w1247]
            tunnel: w310 -> [w1249]
            tunnel: w308 -> [w1248]
            tunnel: w283 -> [w1241]
            tunnel: w281 -> [w1240]
            tunnel: w259 -> [w1239]
            tunnel: w256 -> [w1238]
            tunnel: w253 -> [w1237]
            tunnel: [w1230] -> w144
            tunnel: [w1251] -> w236
            tunnel: [w1245] -> w235
            tunnel: [w1250] -> w234
            tunnel: [w1247] -> w233
            tunnel: [w1249] -> w232
            tunnel: [w1248] -> w231
            tunnel: [w1241] -> w230
            tunnel: [w1240] -> w229
            tunnel: [w1239] -> w228
            tunnel: [w1238] -> w227
            tunnel: [w1237] -> w226
            tunnel: [w1235] -> w225
            tunnel: w224 -> [w1235]
            tunnel: [w1234] -> w167
            tunnel: w166 -> [w1234]
            tunnel: [w1233] -> w165
            tunnel: w164 -> [w1233]
            tunnel: [w1232] -> w163
            tunnel: w162 -> [w1232]
            tunnel: [w1231] -> w161
            tunnel: w160 -> [w1231]
            tunnel: w149 -> [w1229]
            tunnel: [w1228] -> w134
            tunnel: [w1227] -> w133
            tunnel: w127 -> [w1226]
            tunnel: [w1225] -> w124
            tunnel: [w1224] -> w123
            tunnel: w236 -> [w1298]
            tunnel: w235 -> [w1297]
            tunnel: w234 -> [w1296]
            tunnel: w233 -> [w1295]
            tunnel: w232 -> [w1294]
            tunnel: w231 -> [w1293]
            tunnel: w230 -> [w1292]
            tunnel: w229 -> [w1291]
            tunnel: w228 -> [w1290]
            tunnel: w227 -> [w1289]
            tunnel: w226 -> [w1288]
            tunnel: w225 -> [w1281]
            tunnel: [w1298] -> w218
            tunnel: [w1297] -> w217
            tunnel: [w1296] -> w216
            tunnel: [w1295] -> w215
            tunnel: [w1294] -> w214
            tunnel: [w1293] -> w213
            tunnel: [w1292] -> w212
            tunnel: [w1291] -> w211
            tunnel: [w1290] -> w210
            tunnel: [w1289] -> w209
            tunnel: [w1288] -> w208
            tunnel: [w1281] -> w207
            tunnel: [w1280] -> w206
            tunnel: w167 -> [w1278]
            tunnel: w165 -> [w1277]
            tunnel: w163 -> [w1276]
            tunnel: w161 -> [w1275]
            tunnel: [w1278] -> w159
            tunnel: [w1277] -> w157
            tunnel: [w1276] -> w155
            tunnel: [w1275] -> w153
            tunnel: w134 -> [w1274]
            tunnel: w133 -> [w1273]
            tunnel: [w1268] -> w132
            tunnel: w124 -> [w1267]
            tunnel: w123 -> [w1266]
            tunnel: [w1309] -> w254
            tunnel: [w1310] -> w257
            tunnel: [w1311] -> w260
            tunnel: [w1312] -> w282
            tunnel: [w1313] -> w284
            tunnel: [w1314] -> w309
            tunnel: [w1315] -> w311
            tunnel: [w1316] -> w313
            tunnel: [w1317] -> w315
            tunnel: [w1318] -> w317
            tunnel: [w1319] -> w318
            tunnel: w218 -> [w1319]
            tunnel: w217 -> [w1318]
            tunnel: w216 -> [w1317]
            tunnel: w215 -> [w1316]
            tunnel: w214 -> [w1315]
            tunnel: w213 -> [w1314]
            tunnel: w212 -> [w1313]
            tunnel: w211 -> [w1312]
            tunnel: w210 -> [w1311]
            tunnel: w209 -> [w1310]
            tunnel: w208 -> [w1309]
            tunnel: w207 -> [w1305]
            tunnel: w206 -> [w1304]
            tunnel: [w1303] -> w158
            tunnel: w159 -> [w1303]
            tunnel: [w1302] -> w156
            tunnel: w157 -> [w1302]
            tunnel: [w1301] -> w154
            tunnel: w155 -> [w1301]
            tunnel: [w1300] -> w152
            tunnel: w153 -> [w1300]
            tunnel: [w1299] -> w146
            tunnel: w132 -> [w1299]
            frame #0 {
              n18 = Tick Count (ms)() -> (millisecond timer value=w348:u32)
            }
            frame #1 {
              n19 = while {
                tunnel: w380 -> [w387]
                tunnel: [w386] -> w379
                tunnel: [w385] -> w378
                tunnel: w366 -> [w383]
                stop <- w388 stop-if-true
                (unwired) "Daniel Schuster (geb. 20.03.1988)"
                n20 = event shown="[11] \"Write to File\": Value Change" {
                  selector: _ -> [_ _ _ _ _ _ _ _ _ _ _ _]
                  dyn-events: _ -> [_ _ _ _ _ _ _ _ _ _ _ _]
                  timeout: 1 -> [_ _ _ _ _ _ _ _ _ _ _ _]
                  tunnel: [TRUE ("Set Gauge to Zero") w396 w445 w466 w492 w527 w583 w634 w713 w784 "Set Gauge to Zero" _] -> w388
                  tunnel: w387 -> [w392 w395 w442 w464 w488 w526 w579 w632 w711 w782 w859 w881]
                  tunnel: [w391 w394 w441 w463 w490 w524 w581 w631 w710 w781 w858 w880] -> w386
                  tunnel: [w390 w393 w440 w462 w489 w525 w580 w630 w709 w780 w857 w879] -> w385
                  tunnel: w383 -> [_ _ _ _ _ _ _ _ _ _ w855 _]
                  event Timeout {
                    n21 = event-data() -> ()  [unwired: 1 in, 1 out]
                    n22 = Unbundle(w392) -> ("VISA resource name out"=w391:refnum<visa-resource-name>, "error out"=w390:errorcluster)  [unwired: 2 out]
                  }
                  event "Setpoint\n START": Value Change {
                    n23 = event-data() -> ()  [unwired: 1 in, 1 out]
                    n24 = stacked-sequence {
                      tunnel: w395 -> [_ w402 _]
                      tunnel: [_ w401 _] -> w393
                      tunnel: [_ w400 _] -> w394
                      frame #0 {
                        n25 = property on="Setpoint\n START" class="Bool"("Blinking"=TRUE) -> ()  [unwired: 2 in, 2 out]
                        n26 = property on="ON" class="Bool (strict)"("Blinking"=FALSE) -> ()  [unwired: 2 in, 2 out]
                      }
                      frame #1 {
                        n27 = for {
                          N: 2 -> [_]
                          tunnel: w402 -> [w406]
                          tunnel: [w405] -> w401
                          tunnel: [w404] -> w400
                          i -> [w408]
                          n28 = flat-sequence {
                            tunnel: [w411] -> w407
                            tunnel: w408 -> [w410]
                            tunnel: [w429] -> w409
                            tunnel: w407 -> [w428]
                            tunnel: w406 -> [w430]
                            tunnel: [w427] -> w405
                            tunnel: [w426] -> w404
                            tunnel: w409 -> [w436]
                            tunnel: w408 -> [w435]
                            frame #0 {
                              n29 = case shown="0, Default" w410 {
                                tunnel: [w420 w422] -> w411
                                frame 0, Default {
                                n30 = Multiply(x=10.0, y="SP 1 shall be (°C)") -> (x*y=w417:dbl)
                                n31 = local read "RAM"() -> (w415:bool)
                                n32 = Number To Hexadecimal String(1:i16 5 ("width (-)"), 2:w417) -> (0:w419:string)
                                n33 = Select(t="*P012", s=w415, f="*P012") -> (s? t:f=w412:string)
                                n34 = Concatenate Strings(w412, w419) -> (w420:string)
                                }
                                frame 1 {
                                n35 = local read "RAM"() -> (w425:bool)
                                n36 = Select(t="*G01", s=w425, f="*R01") -> (s? t:f=w422:string)
                                }
                              }
                            }
                            frame #1 {
                              n37 = Unbundle(w430) -> ("VISA resource name out"=w431:refnum<visa-resource-name>, "error out"=w433:errorcluster, "Delay (ms)"=w432:u32, "Write/\nRead"=w434:bool)
                              n38 = call "I3252_Comm_Interface.vi"("VISA resource name in"=w431, "error in"=w433, "Delay (ms)"=w432, "Write"=w434, "String to Write"=w428, "Read"=w434) -> ("VISA resource name out"=w426:refnum<visa-resource-name>, "error out"=w427:errorcluster, "Read String"=w429:string)  [unwired: 2 in]
                            }
                            frame #2 {
                              n39 = case shown="0, Default" w435 {
                                tunnel: w436 -> [_ w438]
                                frame 0, Default {
                                }
                                frame 1 {
                                n40 = call "I3252_Edit_Setpoint.vi"("Read String"=w438) -> ("Setpoint is"=→"SP 1 is (°C)":dbl)
                                }
                              }
                            }
                          }
                        }
                      }
                      frame #2 {
                        n41 = property on="Setpoint\n START" class="Bool"("Blinking"=FALSE) -> ()  [unwired: 2 in, 2 out]
                      }
                    }
                    n42 = Not(x="Setpoint\n START") -> (.not. x?=w396:bool)
                  }
                  event "Standby": Value Change {
                    n43 = event-data() -> ()  [unwired: 1 in, 1 out]
                    n44 = flat-sequence {
                      tunnel: [w453] -> w443
                      tunnel: w443 -> [w457]
                      tunnel: w442 -> [w456]
                      tunnel: [w455] -> w440
                      tunnel: [w454] -> w441
                      frame #0 {
                        n45 = local read "Standby"() -> (w446:bool)
                        n46 = Select(t=TRUE, s=w446, f=FALSE) -> (s? t:f=w449:bool)
                        n47 = property on="Standby" class="Bool (strict)"("Blinking"=w449) -> ()  [unwired: 2 in, 2 out]
                      }
                      frame #1 {
                        n48 = local read "Standby"() -> (w451:bool)
                        n49 = Select(t="*D03", s=w451, f="*E03") -> (s? t:f=w453:string)
                      }
                      frame #2 {
                        n50 = Unbundle(w456) -> ("VISA resource name out"=w458:refnum<visa-resource-name>, "error out"=w460:errorcluster, "Delay (ms)"=w459:u32, "Write/\nRead"=w461:bool)
                        n51 = call "I3252_Comm_Interface.vi"("VISA resource name in"=w458, "error in"=w460, "Delay (ms)"=w459, "Write"=w461, "String to Write"=w457, "Read"=w461) -> ("VISA resource name out"=w454:refnum<visa-resource-name>, "error out"=w455:errorcluster)  [unwired: 2 in, 1 out]
                      }
                    }
                    n52 = Not(x="Standby") -> (.not. x?=w445:bool)
                  }
                  event "Set Command": Value Change {
                    n53 = event-data() -> ()  [unwired: 1 in, 1 out]
                    n54 = stacked-sequence {
                      tunnel: w464 -> [_ w471 _]
                      tunnel: [_ w470 _] -> w463
                      tunnel: [_ w469 _] -> w462
                      frame #0 {
                        n55 = property on="Set Command" class="Bool"("Blinking"=TRUE) -> ()  [unwired: 2 in, 2 out]
                        n56 = property on="ON" class="Bool (strict)"("Blinking"=FALSE) -> ()  [unwired: 2 in, 2 out]
                      }
                      frame #1 {
                        n57 = flat-sequence {
                          tunnel: [w476] -> w473
                          tunnel: [w479] -> w472
                          tunnel: w473 -> [w480]
                          tunnel: w471 -> [w481]
                          tunnel: [w478] -> w470
                          tunnel: [w477] -> _
                          tunnel: [w477] -> w469
                          tunnel: w472 -> [w486]
                          frame #0 {
                            n58 = Concatenate Strings("*", "Command input") -> (w476:string)
                          }
                          frame #1 {
                            n59 = Unbundle(w481) -> ("VISA resource name out"=w485:refnum<visa-resource-name>, "error out"=w483:errorcluster, "Delay (ms)"=w484:u32, "Write/\nRead"=w482:bool)
                            n60 = call "I3252_Comm_Interface.vi"("VISA resource name in"=w485, "error in"=w483, "Delay (ms)"=w484, "Write"=w482, "String to Write"=w480, "Read"=w482) -> ("VISA resource name out"=w478:refnum<visa-resource-name>, "error out"=w477:errorcluster, "Read String"=w479:string)  [unwired: 2 in]
                          }
                          frame #2 {
                            "Command output" <- w486
                          }
                        }
                      }
                      frame #2 {
                        n61 = property on="Set Command" class="Bool"("Blinking"=FALSE) -> ()  [unwired: 2 in, 2 out]
                      }
                    }
                    n62 = Not(x="Set Command") -> (.not. x?=w466:bool)
                  }
                  event "Reset\nSTOPP": Value Change {
                    n63 = event-data() -> ()  [unwired: 1 in, 1 out]
                    n64 = stacked-sequence {
                      tunnel: [_ w499 _] -> w489
                      tunnel: [_ w498 _] -> w490
                      tunnel: w488 -> [_ w496 _]
                      frame #0 {
                        n65 = property on="Reset\nSTOPP" class="Bool"("Blinking"=TRUE) -> ()  [unwired: 2 in, 2 out]
                        n66 = property on="ON" class="Bool (strict)"("Blinking"=FALSE) -> ()  [unwired: 2 in, 2 out]
                      }
                      frame #1 {
                        n67 = for {
                          N: 2 -> [_]
                          tunnel: [w505] -> w499
                          tunnel: [w504] -> w498
                          tunnel: w496 -> [w503]
                          i -> [w501]
                          n68 = flat-sequence {
                            tunnel: w501 -> [w507]
                            tunnel: [w506] -> w502
                            tunnel: [w512] -> w505
                            tunnel: [w513] -> w504
                            tunnel: w503 -> [w514]
                            tunnel: w502 -> [w511]
                            tunnel: [w510] -> w500
                            tunnel: w501 -> [w520]
                            tunnel: w500 -> [w519]
                            frame #0 {
                              n69 = case shown="0, Default" w507 {
                                tunnel: ["*Z02" "*G01"] -> w506
                                frame 0, Default {
                                }
                                frame 1 {
                                }
                              }
                            }
                            frame #1 {
                              n70 = Unbundle(w514) -> ("VISA resource name out"=w515:refnum<visa-resource-name>, "error out"=w517:errorcluster, "Delay (ms)"=w516:u32, "Write/\nRead"=w518:bool)
                              n71 = call "I3252_Comm_Interface.vi"("VISA resource name in"=w515, "error in"=w517, "Delay (ms)"=w516, "Write"=w518, "String to Write"=w511, "Read"=w518) -> ("VISA resource name out"=w513:refnum<visa-resource-name>, "error out"=w512:errorcluster, "Read String"=w510:string)  [unwired: 2 in]
                            }
                            frame #2 {
                              n72 = case shown="0, Default" w520 {
                                tunnel: w519 -> [_ w522]
                                frame 0, Default {
                                }
                                frame 1 {
                                n73 = call "I3252_Edit_Setpoint.vi"("Read String"=w522) -> ("Setpoint is"=w521:dbl)
                                n74 = local write "SP 1 is (°C)"(w521) -> ()
                                }
                              }
                            }
                          }
                        }
                        n75 = Wait (ms)(milliseconds to wait=u32 4000) -> ()  [unwired: 1 out]
                      }
                      frame #2 {
                        n76 = property on="Reset\nSTOPP" class="Bool"("Blinking"=FALSE) -> ()  [unwired: 2 in, 2 out]
                      }
                    }
                    n77 = Not(x="Reset\nSTOPP") -> (.not. x?=w492:bool)
                  }
                  event "Auto Tune": Value Change {
                    n78 = event-data() -> ()  [unwired: 1 in, 1 out]
                    n79 = stacked-sequence {
                      tunnel: w526 -> [_ w533 w578]
                      tunnel: [_ w532 _] -> w525
                      tunnel: [_ w531 _] -> w524
                      frame #0 {
                        n80 = property on="Auto Tune" class="Bool"("Blinking"=TRUE) -> ()  [unwired: 2 in, 2 out]
                        n81 = property on="ON" class="Bool (strict)"("Blinking"=FALSE) -> ()  [unwired: 2 in, 2 out]
                      }
                      frame #1 {
                        n82 = for {
                          N: 4 -> [_]
                          tunnel: [w538] -> w531
                          tunnel: [w537] -> w532
                          tunnel: w533 -> [w536]
                          i -> [w541]
                          n83 = flat-sequence {
                            tunnel: w541 -> [w543]
                            tunnel: [w542] -> w539
                            tunnel: w539 -> [w558]
                            tunnel: [w557] -> w540
                            tunnel: [w560] -> w538
                            tunnel: [w559] -> w537
                            tunnel: w536 -> [w556]
                            tunnel: w541 -> [w566]
                            tunnel: w540 -> [w565]
                            frame #0 {
                              n84 = case shown="0, Default" w543 {
                                tunnel: ["*V01" w546 "*W0C35" "*Z02"] -> w542
                                frame 0, Default {
                                }
                                frame 1 {
                                n85 = local read "(°C)"() -> (w545:dbl)
                                n86 = Add(x=20.0, y=w545) -> (x+y=w552:dbl)
                                n87 = Multiply(x=10.0, y=w552) -> (x*y=w549:dbl)
                                n88 = Number To Hexadecimal String(1:i16 5 ("width (-)"), 2:w549) -> (0:w548:string)
                                n89 = Concatenate Strings("*W012", w548) -> (w546:string)
                                }
                                frame 2 {
                                # "35 hex = \n00110101 bin"
                                }
                                frame 3 {
                                }
                              }
                            }
                            frame #1 {
                              n90 = Unbundle(w556) -> ("VISA resource name out"=w564:refnum<visa-resource-name>, "error out"=w562:errorcluster, "Delay (ms)"=w563:u32, "Write/\nRead"=w561:bool)
                              n91 = call "I3252_Comm_Interface.vi"("VISA resource name in"=w564, "error in"=w562, "Delay (ms)"=w563, "Write"=w561, "String to Write"=w558, "Read"=w561) -> ("VISA resource name out"=w560:refnum<visa-resource-name>, "error out"=w559:errorcluster, "Read String"=w557:string)  [unwired: 2 in]
                            }
                            frame #2 {
                              n92 = case shown="0, Default" w566 {
                                tunnel: w565 -> [w568]
                                frame 0, Default {
                                n93 = call <vilib>:"Space Constant.vi"() -> ("String"=w571:string)
                                n94 = Search/Split String(string=w568, search string/char (-)=w571) -> (match + rest of string=w570:string)  [unwired: 1 in, 2 out]
                                n95 = Fract/Exp String To Number(use system decimal point (T)=FALSE, string=w570) -> (number=w567:dbl)  [unwired: 2 in, 1 out]
                                n96 = local write "(°C)"(w567) -> ()
                                }
                              }
                            }
                          }
                        }
                        n97 = Wait (ms)(milliseconds to wait=u32 45000) -> ()  [unwired: 1 out]
                      }
                      frame #2 {
                        n98 = Unbundle(w578) -> ("VISA resource name out"=w577:refnum<visa-resource-name>, "error out"=w575:errorcluster, "Delay (ms)"=w576:u32, "Write/\nRead"=w574:bool)
                        n99 = property on="Auto Tune" class="Bool"("Blinking"=FALSE) -> ()  [unwired: 2 in, 2 out]
                        n100 = call "I3252_Comm_Interface.vi"("VISA resource name in"=w577, "error in"=w575, "Delay (ms)"=w576, "Write"=w574, "String to Write"="*W01200000", "Read"=w574) -> ()  [unwired: 2 in, 3 out]
                      }
                    }
                    n101 = Not(x="Auto Tune") -> (.not. x?=w527:bool)
                  }
                  event "Write LOW/HI": Value Change {
                    n102 = event-data() -> ()  [unwired: 1 in, 1 out]
                    n103 = stacked-sequence {
                      tunnel: [_ w588 _] -> w581
                      tunnel: [_ w587 _] -> w580
                      tunnel: w579 -> [_ w586 _]
                      frame #0 {
                        n104 = property on="Write LOW/HI" class="Bool"("Blinking"=TRUE) -> ()  [unwired: 2 in, 2 out]
                        n105 = property on="ON" class="Bool (strict)"("Blinking"=FALSE) -> ()  [unwired: 2 in, 2 out]
                      }
                      frame #1 {
                        n106 = for {
                          N: 4 -> [_]
                          tunnel: [w592] -> w588
                          tunnel: [w591] -> w587
                          tunnel: w586 -> [w590]
                          i -> [w594]
                          n107 = flat-sequence {
                            tunnel: w594 -> [w596]
                            tunnel: [w597] -> w593
                            tunnel: w593 -> [w611]
                            tunnel: [w612] -> w595
                            tunnel: [w614] -> w592
                            tunnel: [w613] -> w591
                            tunnel: w590 -> [w610]
                            tunnel: w595 -> [w620]
                            tunnel: w594 -> [w619]
                            frame #0 {
                              n108 = case shown="1" w596 {
                                tunnel: [w599 w605 "*R27" "*R28"] -> w597
                                frame 0, Default {
                                n109 = Number To Hexadecimal String(1:i16 2 ("width (-)"), 2:"% LOW Sollwert") -> (0:w600:string)
                                n110 = Concatenate Strings("*W27", w600) -> (w599:string)
                                }
                                frame 1 {
                                n111 = Number To Hexadecimal String(1:i16 2 ("width (-)"), 2:"% High Sollwert") -> (0:w606:string)
                                n112 = Concatenate Strings("*W28", w606) -> (w605:string)
                                }
                                frame 2 {
                                }
                                frame 3 {
                                }
                              }
                            }
                            frame #1 {
                              n113 = Unbundle(w610) -> ("VISA resource name out"=w618:refnum<visa-resource-name>, "error out"=w616:errorcluster, "Delay (ms)"=w617:u32, "Write/\nRead"=w615:bool)
                              n114 = call "I3252_Comm_Interface.vi"("VISA resource name in"=w618, "error in"=w616, "Delay (ms)"=w617, "Write"=w615, "String to Write"=w611, "Read"=w615) -> ("VISA resource name out"=w614:refnum<visa-resource-name>, "error out"=w613:errorcluster, "Read String"=w612:string)  [unwired: 2 in]
                            }
                            frame #2 {
                              n115 = case shown="0, Default" w619 {
                                tunnel: w620 -> [_ w624 w628]
                                frame 0, Default {
                                }
                                frame 2 {
                                n116 = String Subset(string=w624, offset (0)=3) -> (substring=w622:string)  [unwired: 1 in]
                                n117 = Hexadecimal String To Number(string=w622) -> (number=→"% LOW Istwert":u32)  [unwired: 2 in, 1 out]
                                }
                                frame 3 {
                                n118 = String Subset(string=w628, offset (0)=3) -> (substring=w626:string)  [unwired: 1 in]
                                n119 = Hexadecimal String To Number(string=w626) -> (number=→"% HIGH Istwert":u32)  [unwired: 2 in, 1 out]
                                }
                              }
                            }
                          }
                        }
                      }
                      frame #2 {
                        n120 = property on="Write LOW/HI" class="Bool"("Blinking"=FALSE) -> ()  [unwired: 2 in, 2 out]
                      }
                    }
                    n121 = Not(x="Write LOW/HI") -> (.not. x?=w583:bool)
                  }
                  event "Set PID": Value Change {
                    n122 = event-data() -> ()  [unwired: 1 in, 1 out]
                    n123 = stacked-sequence {
                      tunnel: w632 -> [_ w639 _]
                      tunnel: [_ w638 _] -> w631
                      tunnel: [_ w637 _] -> w630
                      frame #0 {
                        n124 = property on="Set PID" class="Bool"("Blinking"=TRUE) -> ()  [unwired: 2 in, 2 out]
                        n125 = property on="ON" class="Bool (strict)"("Blinking"=FALSE) -> ()  [unwired: 2 in, 2 out]
                      }
                      frame #1 {
                        n126 = for {
                          N: 6 -> [_]
                          tunnel: w639 -> [w643]
                          tunnel: [w642] -> w638
                          tunnel: [w641] -> w637
                          i -> [w645]
                          n127 = flat-sequence {
                            tunnel: w645 -> [w647]
                            tunnel: [w648] -> w644
                            tunnel: w644 -> [w689]
                            tunnel: [w685] -> w646
                            tunnel: w643 -> [w688]
                            tunnel: [w687] -> w641
                            tunnel: [w686] -> w642
                            tunnel: w646 -> [w695]
                            tunnel: w645 -> [w694]
                            frame #0 {
                              n128 = case shown="0, Default" w647 {
                                tunnel: [w655 w663 w671 w673 w677 w681] -> w648
                                frame 0, Default {
                                n129 = local read "RAM"() -> (w649:bool)
                                n130 = Number To Hexadecimal String(1:i16 4 ("width (-)"), 2:"P (PB1) Sollwert") -> (0:w656:string)
                                n131 = Select(t="*P17", s=w649, f="*W17") -> (s? t:f=w650:string)
                                n132 = Concatenate Strings(w650, w656) -> (w655:string)
                                }
                                frame 1 {
                                n133 = local read "RAM"() -> (w657:bool)
                                n134 = Number To Hexadecimal String(1:i16 4 ("width (-)"), 2:"I ( Reset1) Sollwert") -> (0:w664:string)
                                n135 = Select(t="*P18", s=w657, f="*W18") -> (s? t:f=w659:string)
                                n136 = Concatenate Strings(w659, w664) -> (w663:string)
                                }
                                frame 2 {
                                n137 = local read "RAM"() -> (w666:bool)
                                n138 = Number To Hexadecimal String(1:i16 4 ("width (-)"), 2:"D (Rate) Sollwert") -> (0:w672:string)
                                n139 = Select(t="*P19", s=w666, f="*W19") -> (s? t:f=w667:string)
                                n140 = Concatenate Strings(w667, w672) -> (w671:string)
                                }
                                frame 3 {
                                n141 = local read "RAM"() -> (w676:bool)
                                n142 = Select(t="*G17", s=w676, f="*R17") -> (s? t:f=w673:string)
                                }
                                frame 4 {
                                n143 = local read "RAM"() -> (w680:bool)
                                n144 = Select(t="*G18", s=w680, f="*R18") -> (s? t:f=w677:string)
                                }
                                frame 5 {
                                n145 = local read "RAM"() -> (w684:bool)
                                n146 = Select(t="*G19", s=w684, f="*R19") -> (s? t:f=w681:string)
                                }
                              }
                            }
                            frame #1 {
                              n147 = Unbundle(w688) -> ("VISA resource name out"=w693:refnum<visa-resource-name>, "error out"=w691:errorcluster, "Delay (ms)"=w692:u32, "Write/\nRead"=w690:bool)
                              n148 = call "I3252_Comm_Interface.vi"("VISA resource name in"=w693, "error in"=w691, "Delay (ms)"=w692, "Write"=w690, "String to Write"=w689, "Read"=w690) -> ("VISA resource name out"=w686:refnum<visa-resource-name>, "error out"=w687:errorcluster, "Read String"=w685:string)  [unwired: 2 in]
                            }
                            frame #2 {
                              n149 = case shown="5" w694 {
                                tunnel: w695 -> [_ w699 w703 w707]
                                frame 0, Default {
                                }
                                frame 3 {
                                n150 = String Subset(string=w699, offset (0)=3) -> (substring=w697:string)  [unwired: 1 in]
                                n151 = Hexadecimal String To Number(string=w697) -> (number=→"P (PB1) Istwert":u32)  [unwired: 2 in, 1 out]
                                }
                                frame 4 {
                                n152 = String Subset(string=w703, offset (0)=3) -> (substring=w701:string)  [unwired: 1 in]
                                n153 = Hexadecimal String To Number(string=w701) -> (number=→"I ( Reset1) Istwert":u32)  [unwired: 2 in, 1 out]
                                }
                                frame 5 {
                                n154 = String Subset(string=w707, offset (0)=3) -> (substring=w705:string)  [unwired: 1 in]
                                n155 = Hexadecimal String To Number(string=w705) -> (number=→"D (Rate) IstWert":u32)  [unwired: 2 in, 1 out]
                                }
                              }
                            }
                          }
                        }
                      }
                      frame #2 {
                        n156 = property on="Set PID" class="Bool"("Blinking"=FALSE) -> ()  [unwired: 2 in, 2 out]
                      }
                    }
                    n157 = Not(x="Set PID") -> (.not. x?=w634:bool)
                  }
                  event "Get Values": Value Change {
                    n158 = event-data() -> ()  [unwired: 1 in, 1 out]
                    n159 = stacked-sequence {
                      tunnel: w711 -> [_ w718 _]
                      tunnel: [_ w717 _] -> w710
                      tunnel: [_ w716 _] -> w709
                      frame #0 {
                        n160 = property on="Get Values" class="Bool"("Blinking"=TRUE) -> ()  [unwired: 2 in, 2 out]
                        n161 = property on="ON" class="Bool (strict)"("Blinking"=FALSE) -> ()  [unwired: 2 in, 2 out]
                      }
                      frame #1 {
                        n162 = for {
                          N: 6 -> [_]
                          tunnel: w718 -> [w722]
                          tunnel: [w721] -> w717
                          tunnel: [w720] -> w716
                          i -> [w724]
                          n163 = flat-sequence {
                            tunnel: w724 -> [w726]
                            tunnel: [w727] -> w723
                            tunnel: w723 -> [w749]
                            tunnel: [w750] -> w725
                            tunnel: w722 -> [w748]
                            tunnel: [w747] -> w720
                            tunnel: [w746] -> w721
                            tunnel: w725 -> [w756]
                            tunnel: w724 -> [w755]
                            frame #0 {
                              n164 = case shown="0, Default" w726 {
                                tunnel: [w730 w734 w738 "*R27" "*R28" w744] -> w727
                                frame 0, Default {
                                n165 = local read "RAM"() -> (w731:bool)
                                n166 = Select(t="*G17", s=w731, f="*R17") -> (s? t:f=w730:string)
                                }
                                frame 1 {
                                n167 = local read "RAM"() -> (w735:bool)
                                n168 = Select(t="*G18", s=w735, f="*R18") -> (s? t:f=w734:string)
                                }
                                frame 2 {
                                n169 = local read "RAM"() -> (w739:bool)
                                n170 = Select(t="*G19", s=w739, f="*R19") -> (s? t:f=w738:string)
                                }
                                frame 3 {
                                }
                                frame 4 {
                                }
                                frame 5 {
                                n171 = local read "RAM"() -> (w745:bool)
                                n172 = Select(t="*G01", s=w745, f="*R01") -> (s? t:f=w744:string)
                                }
                              }
                            }
                            frame #1 {
                              n173 = Unbundle(w748) -> ("VISA resource name out"=w754:refnum<visa-resource-name>, "error out"=w752:errorcluster, "Delay (ms)"=w753:u32, "Write/\nRead"=w751:bool)
                              n174 = call "I3252_Comm_Interface.vi"("VISA resource name in"=w754, "error in"=w752, "Delay (ms)"=w753, "Write"=w751, "String to Write"=w749, "Read"=w751) -> ("VISA resource name out"=w746:refnum<visa-resource-name>, "error out"=w747:errorcluster, "Read String"=w750:string)  [unwired: 2 in]
                            }
                            frame #2 {
                              n175 = case shown="0, Default" w755 {
                                tunnel: w756 -> [w758 w762 w766 w770 w774 w778]
                                frame 0, Default {
                                n176 = String Subset(string=w758, offset (0)=3) -> (substring=w759:string)  [unwired: 1 in]
                                n177 = Hexadecimal String To Number(string=w759) -> (number=w757:u32)  [unwired: 2 in, 1 out]
                                n178 = local write "P (PB1) Sollwert"(w757) -> ()
                                n179 = local write "P (PB1) Istwert"(w757) -> ()
                                }
                                frame 1 {
                                n180 = String Subset(string=w762, offset (0)=3) -> (substring=w763:string)  [unwired: 1 in]
                                n181 = Hexadecimal String To Number(string=w763) -> (number=w761:u32)  [unwired: 2 in, 1 out]
                                n182 = local write "I ( Reset1) Sollwert"(w761) -> ()
                                n183 = local write "I ( Reset1) Istwert"(w761) -> ()
                                }
                                frame 2 {
                                n184 = String Subset(string=w766, offset (0)=3) -> (substring=w767:string)  [unwired: 1 in]
                                n185 = Hexadecimal String To Number(string=w767) -> (number=w765:u32)  [unwired: 2 in, 1 out]
                                n186 = local write "D (Rate) Sollwert"(w765) -> ()
                                n187 = local write "D (Rate) IstWert"(w765) -> ()
                                }
                                frame 3 {
                                n188 = String Subset(string=w770, offset (0)=3) -> (substring=w771:string)  [unwired: 1 in]
                                n189 = Hexadecimal String To Number(string=w771) -> (number=w769:u32)  [unwired: 2 in, 1 out]
                                n190 = local write "% LOW Istwert"(w769) -> ()
                                n191 = local write "% LOW Sollwert"(w769) -> ()
                                }
                                frame 4 {
                                n192 = String Subset(string=w774, offset (0)=3) -> (substring=w775:string)  [unwired: 1 in]
                                n193 = Hexadecimal String To Number(string=w775) -> (number=w773:u32)  [unwired: 2 in, 1 out]
                                n194 = local write "% High Sollwert"(w773) -> ()
                                n195 = local write "% HIGH Istwert"(w773) -> ()
                                }
                                frame 5 {
                                n196 = call "I3252_Edit_Setpoint.vi"("Read String"=w778) -> ("Setpoint is"=w777:dbl)
                                n197 = local write "SP 1 is (°C)"(w777) -> ()
                                }
                              }
                            }
                          }
                        }
                      }
                      frame #2 {
                        n198 = property on="Get Values" class="Bool"("Blinking"=FALSE) -> ()  [unwired: 2 in, 2 out]
                      }
                    }
                    n199 = Not(x="Get Values") -> (.not. x?=w713:bool)
                  }
                  event "RAM": Value Change {
                    n200 = event-data() -> ()  [unwired: 1 in, 1 out]
                    n201 = stacked-sequence {
                      tunnel: w782 -> [_ w789 _]
                      tunnel: [_ w788 _] -> w781
                      tunnel: [_ w787 _] -> w780
                      frame #0 {
                        n202 = property on="RAM" class="Bool (strict)"("Blinking"=TRUE) -> ()  [unwired: 2 in, 2 out]
                        n203 = property on="ON" class="Bool (strict)"("Blinking"=FALSE) -> ()  [unwired: 2 in, 2 out]
                      }
                      frame #1 {
                        n204 = for {
                          N: 6 -> [_]
                          tunnel: w789 -> [w793]
                          tunnel: [w792] -> w788
                          tunnel: [w791] -> w787
                          i -> [w795]
                          n205 = flat-sequence {
                            tunnel: w795 -> [w797]
                            tunnel: [w798] -> w794
                            tunnel: w794 -> [w817]
                            tunnel: [w818] -> w796
                            tunnel: w793 -> [w821]
                            tunnel: [w820] -> w791
                            tunnel: [w819] -> w792
                            tunnel: w796 -> [w827]
                            tunnel: w795 -> [w826]
                            frame #0 {
                              n206 = case shown="0, Default" w797 {
                                tunnel: [w801 w805 w809 "*R27" "*R28" w815] -> w798
                                frame 0, Default {
                                n207 = local read "RAM"() -> (w802:bool)
                                n208 = Select(t="*G17", s=w802, f="*R17") -> (s? t:f=w801:string)
                                }
                                frame 1 {
                                n209 = local read "RAM"() -> (w806:bool)
                                n210 = Select(t="*G18", s=w806, f="*R18") -> (s? t:f=w805:string)
                                }
                                frame 2 {
                                n211 = local read "RAM"() -> (w810:bool)
                                n212 = Select(t="*G19", s=w810, f="*R19") -> (s? t:f=w809:string)
                                }
                                frame 3 {
                                }
                                frame 4 {
                                }
                                frame 5 {
                                n213 = local read "RAM"() -> (w816:bool)
                                n214 = Select(t="*G01", s=w816, f="*R01") -> (s? t:f=w815:string)
                                }
                              }
                            }
                            frame #1 {
                              n215 = Unbundle(w821) -> ("VISA resource name out"=w825:refnum<visa-resource-name>, "error out"=w823:errorcluster, "Delay (ms)"=w824:u32, "Write/\nRead"=w822:bool)
                              n216 = call "I3252_Comm_Interface.vi"("VISA resource name in"=w825, "error in"=w823, "Delay (ms)"=w824, "Write"=w822, "String to Write"=w817, "Read"=w822) -> ("VISA resource name out"=w819:refnum<visa-resource-name>, "error out"=w820:errorcluster, "Read String"=w818:string)  [unwired: 2 in]
                            }
                            frame #2 {
                              n217 = case shown="0, Default" w826 {
                                tunnel: w827 -> [w829 w833 w837 w841 w845 w849]
                                frame 0, Default {
                                n218 = String Subset(string=w829, offset (0)=3) -> (substring=w830:string)  [unwired: 1 in]
                                n219 = Hexadecimal String To Number(string=w830) -> (number=w828:u32)  [unwired: 2 in, 1 out]
                                n220 = local write "P (PB1) Sollwert"(w828) -> ()
                                n221 = local write "P (PB1) Istwert"(w828) -> ()
                                }
                                frame 1 {
                                n222 = String Subset(string=w833, offset (0)=3) -> (substring=w834:string)  [unwired: 1 in]
                                n223 = Hexadecimal String To Number(string=w834) -> (number=w832:u32)  [unwired: 2 in, 1 out]
                                n224 = local write "I ( Reset1) Sollwert"(w832) -> ()
                                n225 = local write "I ( Reset1) Istwert"(w832) -> ()
                                }
                                frame 2 {
                                n226 = String Subset(string=w837, offset (0)=3) -> (substring=w838:string)  [unwired: 1 in]
                                n227 = Hexadecimal String To Number(string=w838) -> (number=w836:u32)  [unwired: 2 in, 1 out]
                                n228 = local write "D (Rate) IstWert"(w836) -> ()
                                n229 = local write "D (Rate) Sollwert"(w836) -> ()
                                }
                                frame 3 {
                                n230 = String Subset(string=w841, offset (0)=3) -> (substring=w842:string)  [unwired: 1 in]
                                n231 = Hexadecimal String To Number(string=w842) -> (number=w840:u32)  [unwired: 2 in, 1 out]
                                n232 = local write "% LOW Istwert"(w840) -> ()
                                n233 = local write "% LOW Sollwert"(w840) -> ()
                                }
                                frame 4 {
                                n234 = String Subset(string=w845, offset (0)=3) -> (substring=w846:string)  [unwired: 1 in]
                                n235 = Hexadecimal String To Number(string=w846) -> (number=w844:u32)  [unwired: 2 in, 1 out]
                                n236 = local write "% HIGH Istwert"(w844) -> ()
                                n237 = local write "% High Sollwert"(w844) -> ()
                                }
                                frame 5 {
                                n238 = call "I3252_Edit_Setpoint.vi"("Read String"=w849) -> ("Setpoint is"=w848:dbl)
                                n239 = local write "SP 1 is (°C)"(w848) -> ()
                                }
                              }
                            }
                          }
                        }
                      }
                      frame #2 {
                        n240 = property on="RAM" class="Bool (strict)"("Blinking"=FALSE) -> ()  [unwired: 2 in, 2 out]
                      }
                    }
                    n241 = Not(x="RAM") -> (.not. x?=w784:bool)
                  }
                  event "Set Gauge to Zero": Value Change {
                    n242 = event-data() -> ()  [unwired: 1 in, 1 out]
                    n243 = flat-sequence {
                      tunnel: w855 -> [w860]
                      tunnel: [w860] -> w854
                      tunnel: w854 -> [w862]
                      tunnel: [w866] -> w853
                      tunnel: [w865] -> w852
                      tunnel: [w862] -> w851
                      tunnel: w853 -> [w872]
                      tunnel: w852 -> [w871]
                      tunnel: w851 -> [w867]
                      frame #0 {
                        n244 = property on="Set Gauge to Zero" class="Bool"("Blinking"=TRUE) -> ()  [unwired: 2 in, 2 out]
                      }
                      frame #1 {
                        w863 = 0 items=["sensor 1", "sensor 2", "test"] ("Sensor Nr.:")
                        n245 = call "DUAL GAUGE-Get Pressure,Status.vi"("Sensor Nr.:"=w863, "Referenz in"=w862) -> ("Pressure"=w866:dbl)  [unwired: 6 in, 3 out]
                        n246 = call "DUAL GAUGE-Offset display.vi"("W/R"=FALSE, "Referenz in"=w862) -> ("Sensor 1 Get"=w865:dbl)  [unwired: 6 in, 3 out]
                      }
                      frame #2 {
                        n247 = Add(x=w872, y=w871) -> (x+y=w868:dbl)
                        n248 = call "DUAL GAUGE-Offset display.vi"("W/R"=TRUE, "Sensor 1 Set"=w868, "Referenz in"=w867) -> ("Sensor 1 Get"=→"Current Offset (mbar)":dbl)  [unwired: 5 in, 3 out]
                      }
                      frame #3 {
                        n249 = property on="Set Gauge to Zero" class="Bool"("Blinking"=TRUE) -> ()  [unwired: 2 in, 2 out]
                      }
                    }
                    n250 = Unbundle(w859) -> ("VISA resource name out"=w858:refnum<visa-resource-name>, "error out"=w857:errorcluster)  [unwired: 2 out]
                  }
                  event "Write to File": Value Change {
                    n251 = event-data() -> ("NewVal"=w878:bool)  [unwired: 1 in]
                    n252 = Unbundle(w881) -> ("VISA resource name out"=w880:refnum<visa-resource-name>, "error out"=w879:errorcluster)  [unwired: 2 out]
                    n253 = local read "File Path"() -> (w874:path)
                    n254 = case shown="True" w878 {
                      tunnel: w874 -> [_ w886]
                      tunnel: "User" -> [_ w885]
                      tunnel: "Sample" -> [_ w884]
                      tunnel: [path "" ("File Path") w883] -> w875
                      frame False {
                      }
                      frame True {
                        n255 = call "Header.vi"("Sample"=w884, "User"=w885, "File Path"=w886) -> ("File Path"=w883:path)
                      }
                    }
                    n256 = local write "File Path"(w875) -> ()
                  }
                }
              }
              n257 = Bundle(cluster=w380, "VISA resource name out"=w379, "error out"=w378) -> (w377:T7)  [unwired: 2 in]
            }
            frame #2 {
            }
            frame #3 {
              (unwired) "Daniel Schuster (geb. 20.03.1988)"
              n258 = node-c288(w939) -> (w948:T3)  [unwired: 2 in]
              n259 = node-c288(w954) -> (w957:T3)  [unwired: 2 in]
              n260 = node-c288(w944) -> (w946:T3)  [unwired: 2 in]
              n261 = node-c288(w953) -> (w961:T3)  [unwired: 2 in]
              n262 = timed-sequence {
                timing: w948 -> [_]
                timing-out: [_] -> w947
                tunnel: w923 -> [w1004]
                tunnel: w922 -> [w1000]
                tunnel: [w1003] -> w915
                tunnel: w914 -> [w1002]
                tunnel: w913 -> [w1001]
                tunnel: [w999] -> w912
                tunnel: [w998] -> w911
                tunnel: [w997] -> w909
                n263 = timed-flat-sequence {
                  tunnel: w1004 -> [w1013]
                  tunnel: [w1012] -> w1003
                  tunnel: w1002 -> [w1011]
                  tunnel: w1001 -> [w1010]
                  tunnel: w1000 -> [w1009]
                  tunnel: [w1007] -> w999
                  tunnel: [w1006] -> w998
                  tunnel: [w1005] -> w997
                  n264 = node-c288() -> ()  [unwired: 1 in, 1 out]
                  n265 = case shown="True" "ON (TPG 2)" {
                    tunnel: w1009 -> [w1018 w1024]
                    tunnel: w1010 -> [w1017 w1023]
                    tunnel: [w1016 w1022] -> w1006
                    tunnel: [w1015 w1021] -> w1005
                    frame False {
                      w1019 = 0.0 ("Pressure")
                      n266 = property on="ON (TPG 2)" class="Bool (strict)"("Blinking"=FALSE) -> ()  [unwired: 2 in, 2 out]
                      n267 = Bundle("Pressure"=w1019, "Pressure"=w1019) -> (w1016:cluster{"Pressure":dbl, "Pressure":dbl})  [unwired: 1 in]
                      n268 = Bundle("TPG 2 COM"=w1018, "error out"=w1017) -> (w1015:T8)  [unwired: 1 in]
                    }
                    frame True {
                      n269 = stacked-sequence {
                        tunnel: w1024 -> [_ w1037]
                        tunnel: [_ w1033] -> w1022
                        tunnel: [_ w1029] -> w1021
                        tunnel: w1023 -> [_ w1026]
                        frame #0 {
                          n270 = property on="ON (TPG 2)" class="Bool (strict)"("Blinking"=TRUE) -> ()  [unwired: 2 in, 2 out]
                        }
                        frame #1 {
                          n271 = call "PresureGetSubVI.vi"("COM in"=w1037, "Fehler (Eingang)"=w1026) -> ("Status Gauge#1"=→"Status Gauge 2#1":i32, "Status Gauge#2"=→"Status Gauge 2#2":i32, "COM out"=w1030:refnum<visa-resource-name>, "Pressure Gauge#1"=w1031:dbl, "Pressure Gauge#2"=w1034:dbl, "Cluster (Ausgang)"=w1027:errorcluster)  [unwired: 12 in]
                          "Pressure Gauge 2#1" <- w1031
                          "Pressure Gauge 2#2" <- w1034
                          n272 = Bundle("COM out"=w1030, "Cluster (Ausgang)"=w1027) -> (w1029:T9)  [unwired: 1 in]
                          n273 = Unbundle(w1027) -> ("status"=w1028:bool, "code"=w1032:i32)  [unwired: 1 out]
                          n274 = Bundle("status"=w1028, "code"=w1032) -> ()  [unwired: 1 in, 1 out]
                          n275 = Bundle("Pressure Gauge#1"=w1031, "Pressure Gauge#2"=w1034) -> (w1033:T10)  [unwired: 1 in]
                        }
                      }
                    }
                  }
                  n276 = case shown="True" "ON (TPG 1)" {
                    tunnel: w1013 -> [w1041 w1047]
                    tunnel: [w1040 w1046] -> w1012
                    tunnel: w1011 -> [w1039 w1045]
                    tunnel: [w1038 w1044] -> w1007
                    frame False {
                      w1042 = 0.0 ("Pressure")
                      n277 = property on="ON (TPG 1)" class="Bool (strict)"("Blinking"=FALSE) -> ()  [unwired: 2 in, 2 out]
                      n278 = Bundle("Pressure"=w1042, "Pressure"=w1042) -> (w1038:cluster{"Pressure":dbl, "Pressure":dbl})  [unwired: 1 in]
                      n279 = Bundle("TPG 1 COM"=w1041, "error out"=w1039) -> (w1040:T11)  [unwired: 1 in]
                    }
                    frame True {
                      n280 = stacked-sequence {
                        tunnel: w1047 -> [_ w1060]
                        tunnel: [_ w1053] -> w1046
                        tunnel: w1045 -> [_ w1050]
                        tunnel: [_ w1049] -> w1044
                        frame #0 {
                          n281 = property on="ON (TPG 1)" class="Bool (strict)"("Blinking"=TRUE) -> ()  [unwired: 2 in, 2 out]
                        }
                        frame #1 {
                          n282 = call "PresureGetSubVI.vi"("COM in"=w1060, "Fehler (Eingang)"=w1050) -> ("Status Gauge#1"=→"Status Gauge 1#1":i32, "Status Gauge#2"=→"Status Gauge 1#2":i32, "COM out"=w1054:refnum<visa-resource-name>, "Pressure Gauge#1"=w1055:dbl, "Pressure Gauge#2"=w1057:dbl, "Cluster (Ausgang)"=w1051:errorcluster)  [unwired: 12 in]
                          "Pressure Gauge 1#1" <- w1055
                          "Pressure Gauge 1#2" <- w1057
                          n283 = Bundle("COM out"=w1054, "Cluster (Ausgang)"=w1051) -> (w1053:T9)  [unwired: 1 in]
                          n284 = Unbundle(w1051) -> ("status"=w1052:bool, "code"=w1056:i32)  [unwired: 1 out]
                          n285 = Bundle("status"=w1052, "code"=w1056) -> ()  [unwired: 1 in, 1 out]
                          n286 = Bundle("Pressure Gauge#1"=w1055, "Pressure Gauge#2"=w1057) -> (w1049:T10)  [unwired: 1 in]
                        }
                      }
                    }
                  }
                  n287 = node-c288() -> ()  [unwired: 1 in, 1 out]
                }
              }
              n288 = timed-sequence {
                timing: w957 -> [_]
                timing-out: [_] -> w956
                tunnel: w955 -> [w1070]
                tunnel: [w1069] -> w950
                tunnel: [w1068] -> w949
                tunnel: [w1067] -> w936
                n289 = timed-flat-sequence {
                  tunnel: w1070 -> [w1074]
                  tunnel: [w1073] -> w1069
                  tunnel: [w1072] -> w1068
                  tunnel: [w1071] -> w1067
                  n290 = node-c288() -> ()  [unwired: 1 in, 1 out]
                  n291 = case shown="True" "ON" {
                    tunnel: w1074 -> [w1078 w1083]
                    tunnel: [w1077 w1082] -> w1073
                    tunnel: [w1076 w1081] -> w1072
                    tunnel: [_ w1080] -> w1071
                    frame False {
                      n292 = Unbundle(w1078) -> ("VISA resource name out"=w1077:refnum<visa-resource-name>, "error out"=w1076:errorcluster)  [unwired: 2 out]
                      n293 = property on="ON" class="Bool (strict)"("Blinking"=FALSE) -> ()  [unwired: 2 in, 2 out]
                    }
                    frame True {
                      n294 = stacked-sequence {
                        tunnel: w1083 -> [_ w1088]
                        tunnel: [_ w1087] -> w1082
                        tunnel: [_ w1086] -> w1081
                        tunnel: [_ w1085] -> w1080
                        frame #0 {
                          n295 = property on="ON" class="Bool (strict)"("Blinking"=TRUE) -> ()  [unwired: 2 in, 2 out]
                        }
                        frame #1 {
                          n296 = Unbundle(w1088) -> ("VISA resource name out"=w1092:refnum<visa-resource-name>, "error out"=w1090:errorcluster, "Delay (ms)"=w1091:u32, "Write/\nRead"=w1089:bool)
                          n297 = call "I3252_Comm_Interface.vi"("VISA resource name in"=w1092, "error in"=w1090, "Delay (ms)"=w1091, "Write"=w1089, "String to Write"="*V01", "Read"=w1089) -> ("VISA resource name out"=w1087:refnum<visa-resource-name>, "error out"=w1086:errorcluster, "Read String"=w1085:string)  [unwired: 2 in]
                        }
                      }
                    }
                  }
                  n298 = node-c288() -> ()  [unwired: 1 in, 1 out]
                }
              }
              n299 = timed-sequence {
                timing: w946 -> [_]
                timing-out: [_] -> w945
                tunnel: w943 -> [w966]
                tunnel: w942 -> [w965]
                tunnel: [w964] -> w940
                tunnel: [w963] -> w941
                tunnel: [w962] -> w937
                n300 = timed-flat-sequence {
                  tunnel: w966 -> [w971]
                  tunnel: w965 -> [w970]
                  tunnel: [w969] -> w964
                  tunnel: [w968] -> w963
                  tunnel: [w967] -> w962
                  n301 = node-c288() -> ()  [unwired: 1 in, 1 out]
                  n302 = case shown="False" "ON" {
                    tunnel: w971 -> [w975 w981]
                    tunnel: w970 -> [w976 w980]
                    tunnel: [w975 w979] -> w969
                    tunnel: [w976 w978] -> w968
                    tunnel: [0.0 ("Reading") w977] -> w967
                    frame False {
                      n303 = property on="ON" class="Bool (strict)"("Blinking"=FALSE) -> ()  [unwired: 2 in, 2 out]
                    }
                    frame True {
                      n304 = stacked-sequence {
                        tunnel: w981 -> [_ w988]
                        tunnel: w980 -> [_ w987]
                        tunnel: [_ w986] -> w979
                        tunnel: [_ w985] -> w978
                        tunnel: [_ w983] -> w977
                        frame #0 {
                          n305 = property on="ON" class="Bool (strict)"("Blinking"=TRUE) -> ()  [unwired: 2 in, 2 out]
                        }
                        frame #1 {
                          n306 = call "VC840_Read.vi"("error in (no error)"=w987, "VISA resource name"=w988) -> ("error out"=w985:errorcluster, "Unit"=→"Unit 2":string, "Reading"=w983:dbl, "VISA resource name out"=w986:refnum<visa-resource-name>, "Status"=→"Status 2":T2, "Mode"=→"Mode 2":enum16{"?", "Diode", "Beep", "DC", "AC"})  [unwired: 4 out]
                          "Reading 2" <- w983
                        }
                      }
                    }
                  }
                  n307 = node-c288() -> ()  [unwired: 1 in, 1 out]
                }
              }
              n308 = timed-sequence {
                timing: w961 -> [_]
                timing-out: [_] -> w960
                tunnel: w959 -> [w1104]
                tunnel: w958 -> [w1103]
                tunnel: [w1102] -> w952
                tunnel: [w1101] -> w951
                tunnel: [w1100] -> w938
                n309 = timed-flat-sequence {
                  tunnel: w1104 -> [w1109]
                  tunnel: w1103 -> [w1108]
                  tunnel: [w1107] -> w1102
                  tunnel: [w1106] -> w1101
                  tunnel: [w1105] -> w1100
                  n310 = node-c288() -> ()  [unwired: 1 in, 1 out]
                  n311 = case shown="True" "ON" {
                    tunnel: w1109 -> [w1113 w1119]
                    tunnel: w1108 -> [w1114 w1118]
                    tunnel: [w1113 w1117] -> w1107
                    tunnel: [w1114 w1116] -> w1106
                    tunnel: [0.0 ("Reading") w1115] -> w1105
                    frame False {
                      n312 = property on="ON" class="Bool (strict)"("Blinking"=FALSE) -> ()  [unwired: 2 in, 2 out]
                    }
                    frame True {
                      n313 = stacked-sequence {
                        tunnel: w1119 -> [_ w1126]
                        tunnel: w1118 -> [_ w1125]
                        tunnel: [_ w1124] -> w1117
                        tunnel: [_ w1123] -> w1116
                        tunnel: [_ w1121] -> w1115
                        frame #0 {
                          n314 = property on="ON" class="Bool (strict)"("Blinking"=TRUE) -> ()  [unwired: 2 in, 2 out]
                        }
                        frame #1 {
                          n315 = call "VC840_Read.vi"("error in (no error)"=w1125, "VISA resource name"=w1126) -> ("error out"=w1123:errorcluster, "Unit"=→"Unit 1":string, "Reading"=w1121:dbl, "VISA resource name out"=w1124:refnum<visa-resource-name>, "Status"=→"Status 1":T2, "Mode"=→"Mode 1":enum16{"?", "Diode", "Beep", "DC", "AC"})  [unwired: 4 out]
                          "Reading 1" <- w1121
                        }
                      }
                    }
                  }
                  n316 = node-c288() -> ()  [unwired: 1 in, 1 out]
                }
              }
              n317 = Tick Count (ms)() -> (millisecond timer value=w924:u32)
              n318 = Subtract(x=w924, y=w929) -> (x-y=w928:u32)
              n319 = Divide(x=w928, y=u32 1000) -> (x/y=w926:dbl)
              n320 = node-c288(w960) -> ()  [unwired: 1 out]
              n321 = node-c288(w945) -> ()  [unwired: 1 out]
              n322 = node-c288(w956) -> ()  [unwired: 1 out]
              n323 = To Double Precision Float(number=w926) -> (double precision float=w930:dbl)
              "current time (s)" <- w930
              n324 = node-c288(w947) -> ()  [unwired: 1 out]
              n325 = Unbundle(w911) -> ("Pressure Gauge#1"=w910:dbl, "Pressure Gauge#2"=w908:dbl)
              "Pressure OpenPort2" <- w908
              "Pressure Pirani 2" <- w910
              n326 = Unbundle(w912) -> ("Pressure Gauge#1"=w921:dbl, "Pressure Gauge#2"=w916:dbl)
              "Pressure Baratron 2" <- w921
              "Pressure FullRange 2" <- w916
            }
            frame #4 {
              n327 = Build Array (concatenate)(w1146, w1150) -> (w1145:dbl[])
              n328 = Build Array (concatenate)(w1149, w1151) -> (w1144:dbl[])
              n329 = Build Array (concatenate)(w1147, w1138) -> (w1142:dbl[])
              n330 = Build Array (concatenate)(w1148, w1139) -> (w1143:dbl[])
              n331 = Greater?(x=w1170, y="Pressure Limit (mbar)") -> (0:w1173:bool)
              n332 = case shown="False" w1173 {
                frame False {
                  n333 = property on="Standby" class="Bool (strict)"("DisabledEnum"=T6."Enabled" ("Disabled")) -> ()  [unwired: 2 in, 2 out]
                }
                frame True {
                  n334 = property on="Standby" class="Bool (strict)"("Val(Sgnl)"=TRUE ("Standby"), "DisabledEnum"=T6."Disabled" ("Disabled")) -> ()  [unwired: 2 in, 2 out]
                }
              }
              n335 = call "Resistivity_Calculation.vi"("Reading 1 (V)"=w1163, "Constant"="Constant", "Thickness (nm)"="Thickness (nm)", "Reading 2 (A)"=w1171) -> ("Resivtivity (Ohm*cm)"=w1155:dbl, "Current"=w1156:dbl, "Voltage"=w1157:dbl)
              "Resistivity (Ohm*cm)" <- w1155
              "Voltage (V)" <- w1157
              "Current (A)" <- w1156
              n336 = call "I3252_Edit_Temperature.vi"("Temp. String"=w1172) -> ("Temp. (°C)"=w1166:dbl)
              "(°C)" <- w1166
              n337 = Build Array (concatenate)(w1168, w1169) -> (w1165:dbl[])
              n338 = Build Array (concatenate)(w1167, w1166) -> (w1153:dbl[])
              n339 = Build Array (concatenate)(w1164, w1157) -> (w1162:dbl[])
              n340 = Build Array (concatenate)(w1161, w1156) -> (w1159:dbl[])
              n341 = Build Array (concatenate)(w1160, w1155) -> (w1158:dbl[])
              n342 = Build Array(w1157, w1156, w1155) -> (w1154:dbl[])
            }
            frame #5 {
              n343 = Bundle(w1201, w1200) -> (→"CMR275 Baratron":cluster{dbl[], dbl[]})  [unwired: 1 in]
              n344 = Bundle(w1201, w1199) -> (→"PKR251 FullRange":cluster{dbl[], dbl[]})  [unwired: 1 in]
              n345 = Bundle(w1201, w1198) -> (→"Pirani (VVP1 Scroll)":cluster{dbl[], dbl[]})  [unwired: 1 in]
              n346 = Bundle(w1201, w1197) -> (→"Pressure OpenPort":cluster{dbl[], dbl[]})  [unwired: 1 in]
              n347 = Bundle(w1201, w1207) -> (→"Thermocouple (Sample holder 1)":cluster{dbl[], dbl[]})  [unwired: 1 in]
              n348 = Bundle(w1201, w1209) -> (→"Voltage":cluster{dbl[], dbl[]})  [unwired: 1 in]
              n349 = Bundle(w1201, w1210) -> (→"Current":cluster{dbl[], dbl[]})  [unwired: 1 in]
              n350 = Bundle(w1201, w1211) -> (→"Resistivity":cluster{dbl[], dbl[]})  [unwired: 1 in]
              n351 = Build Array (concatenate)(w1206, w1216, w1215, w1205, w1192, w1188, w1186) -> (w1223:dbl[])
              "appended array" <- w1223
            }
            frame #6 {
              n352 = Unbundle(w1229) -> ("COM out"=w1228:refnum<visa-resource-name>, "Cluster (Ausgang)"=w1227:errorcluster)
              n353 = Unbundle(w1226) -> ("COM out"=w1225:refnum<visa-resource-name>, "Cluster (Ausgang)"=w1224:errorcluster)
              n354 = case shown="True" "Write to File" {
                tunnel: [_ w1257] -> w1243
                tunnel: "File Path" -> [_ w1255]
                tunnel: w1236 -> [_ w1253]
                frame False {
                  n355 = property on="Write to File" class="Bool (strict)"("Blinking"=FALSE) -> ()  [unwired: 2 in, 2 out]
                }
                frame True {
                  n356 = flat-sequence {
                    tunnel: [w1259] -> w1256
                    tunnel: w1255 -> [w1259]
                    tunnel: [w1258] -> w1254
                    tunnel: w1253 -> [w1258]
                    tunnel: [w1264] -> w1257
                    tunnel: w1256 -> [w1263]
                    tunnel: w1254 -> [w1262]
                    frame #0 {
                      n357 = property on="Write to File" class="Bool (strict)"("Blinking"=TRUE) -> ()  [unwired: 2 in, 2 out]
                    }
                    frame #1 {
                      n358 = call-poly <vilib>:"Write To Spreadsheet File.vi"("format (%.3f)"="%g", "append to file? (new file:F)"=TRUE ("transpose? (no:F)"), "1D data"=w1262, "file path (dialog if empty)"=w1263) -> ("new file path (Not A Path if cancelled)"=w1264:path)  [unwired: 4 in]
                    }
                  }
                }
              }
              n359 = Merge Errors(w1248, w1247, w1245, w1227, w1224) -> (w1246:errorcluster)
              n360 = call <vilib>:"Simple Error Handler.vi"("error in (no error)"=w1246) -> ("error?"=w1230:bool)  [unwired: 4 in, 4 out]
              n361 = local write "File Path"(w1243) -> ()
            }
            frame #7 {
              w1280 = u32 1000 ("y")
              n362 = Tick Count (ms)() -> (millisecond timer value=w1282:u32)
              n363 = Subtract(x=w1282, y=w1281) -> (x-y=w1283:u32)
              n364 = VISA Flush I/O Buffer(VISA resource name=w1274, error in (no error)=w1273) -> (VISA resource name out=w1271:refnum<visa-resource-name>, error out=w1272:errorcluster)  [unwired: 1 in]
              n365 = VISA Flush I/O Buffer(VISA resource name=w1267, error in (no error)=w1266) -> (VISA resource name out=w1270:refnum<visa-resource-name>, error out=w1269:errorcluster)  [unwired: 1 in]
              n366 = Divide(x=w1283, y=w1280) -> (x/y=→"loop time (s)":dbl)
              n367 = Subtract(x="Intervall (s)", y=u32 1) -> (x-y=w1284:u32)
              n368 = Multiply(x=w1284, y=w1280) -> (x*y=w1287:u32)
              n369 = Wait (ms)(milliseconds to wait=w1287) -> ()  [unwired: 1 out]
              n370 = Bundle("COM out"=w1271, "error out"=w1272, "COM out"=w1270, "error out"=w1269) -> (w1268:T12)  [unwired: 1 in]
            }
            frame #8 {
              n371 = Tick Count (ms)() -> (millisecond timer value=w1307:u32)
              n372 = Subtract(x=w1307, y=w1305) -> (x-y=w1306:u32)
              n373 = Divide(x=w1306, y=w1304) -> (x/y=→"data logger intervall (s)":dbl)
            }
          }
          n374 = Exclusive Or(1:"stop", 2:w144) -> (0:w145:bool)
        }
      }
      frame #4 {
        n375 = call "VC840_Close.vi"("error in (no error)"=w1326, "VISA resource name"=w1327) -> ("error out"=w1335:errorcluster)  [unwired: 9 in]
        n376 = call "VC840_Close.vi"("error in (no error)"=w1328, "VISA resource name"=w1329) -> ("error out"=w1333:errorcluster)  [unwired: 9 in]
        n377 = VISA Close(VISA resource name=w1331, error in (no error)=w1330) -> (error out=w1332:errorcluster)
        n378 = Unbundle(w1324) -> ("COM out"=w1323:refnum<visa-resource-name>, "error out"=w1322:errorcluster, "COM out"=w1320:refnum<visa-resource-name>, "error out"=w1321:errorcluster)
        n379 = VISA Close(VISA resource name=w1323, error in (no error)=w1322) -> ()  [unwired: 1 out]
        n380 = VISA Close(VISA resource name=w1320, error in (no error)=w1321) -> ()  [unwired: 1 out]
        n381 = Merge Errors(w1332, w1333, w1335) -> (w1334:errorcluster)
        n382 = call <vilib>:"Simple Error Handler.vi"("error in (no error)"=w1334) -> ("error?"=w1325:bool)  [unwired: 1 in, 7 out]
        n383 = Stop(stop? (T)=w1325) -> ()
      }
    }
  }
